vi "RTK Multiple String Capture Software.vi"() -> ()   [LabVIEW 2010]
uses:
  COM Port Control.ctl
  <vilib>/Utility/sysdir.llb/System Directory Type.ctl
  binary clusters control.ctl
  <vilib>/Instr/_visa.llb/VISA Configure Serial Port (Instr).vi
panel:
  out "shutdown blocker":bool
  in  "Tab Control":T1(tab)
  in  "Update setup":bool
  in  "stop":bool
  in  "Base File Path":path caption="Base File Path (Destination that all RCVR files will be saved in)"
  in  "Time between samples (seconds)":u32=5 min=1 max=600 step=1
  in  "Number of hours To Collect before starting new file":u16=1 min=1 max=24 step=1
  in  "UPDT COM 1":bool
  in  "Use RCVR 1":bool caption="Use RCVR"
  in  "Name of RCVR 1":string="RCVR 1" caption="Name of RCVR"
  in  "COM Port 1":T2={"flow control"=0, "COM Port"="", "parity"=enum."None", "data bits"=8, "baud rate"=9600} {"data bits" min=5 max=8 step=1; "flow control" items=["None", "XON/XOFF", "RTS/CTS", "XON/XOFF & RTS/CTS", "DTR/DSR", "XON/XOFF & DTR/DSR"]}
  out "Last 10 RCVR 1":string[](array[string])
  in  "Name of RCVR 2":string="RCVR 2" caption="Name of RCVR"
  in  "UPDT COM 2":bool
  out "Last 10 RCVR 2":string[](array[string])
  in  "COM Port 2":T2={"flow control"=0, "COM Port"="", "parity"=enum."None", "data bits"=8, "baud rate"=9600} {"data bits" min=5 max=8 step=1; "flow control" items=["None", "XON/XOFF", "RTS/CTS", "XON/XOFF & RTS/CTS", "DTR/DSR", "XON/XOFF & DTR/DSR"]}
  in  "Use RCVR 2":bool caption="Use RCVR"
  in  "Name of RCVR 3":string="RCVR 3" caption="Name of RCVR"
  in  "UPDT COM 3":bool
  out "Last 10 RCVR 3":string[](array[string])
  in  "COM Port 3":T2={"flow control"=0, "COM Port"="", "parity"=enum."None", "data bits"=8, "baud rate"=9600} {"data bits" min=5 max=8 step=1; "flow control" items=["None", "XON/XOFF", "RTS/CTS", "XON/XOFF & RTS/CTS", "DTR/DSR", "XON/XOFF & DTR/DSR"]}
  in  "Use RCVR 3":bool caption="Use RCVR"
  in  "Name of RCVR 4":string="RCVR 4" caption="Name of RCVR"
  in  "UPDT COM 4":bool
  out "Last 10 RCVR 4":string[](array[string])
  in  "COM Port 4":T2={"flow control"=0, "COM Port"="", "parity"=enum."None", "data bits"=8, "baud rate"=9600} {"data bits" min=5 max=8 step=1; "flow control" items=["None", "XON/XOFF", "RTS/CTS", "XON/XOFF & RTS/CTS", "DTR/DSR", "XON/XOFF & DTR/DSR"]}
  in  "Use RCVR 4":bool caption="Use RCVR"
  in  "Name of RCVR 5":string="RCVR 5" caption="Name of RCVR"
  in  "UPDT COM 5":bool
  out "Last 10 RCVR 5":string[](array[string])
  in  "COM Port 5":T2={"flow control"=0, "COM Port"="", "parity"=enum."None", "data bits"=8, "baud rate"=9600} {"data bits" min=5 max=8 step=1; "flow control" items=["None", "XON/XOFF", "RTS/CTS", "XON/XOFF & RTS/CTS", "DTR/DSR", "XON/XOFF & DTR/DSR"]}
  in  "Use RCVR 5":bool caption="Use RCVR"
  in  "Name of RCVR 6":string="RCVR 6" caption="Name of RCVR"
  in  "UPDT COM 6":bool
  out "Last 10 RCVR 6":string[](array[string])
  in  "COM Port 6":T2={"flow control"=0, "COM Port"="", "parity"=enum."None", "data bits"=8, "baud rate"=9600} {"data bits" min=5 max=8 step=1; "flow control" items=["None", "XON/XOFF", "RTS/CTS", "XON/XOFF & RTS/CTS", "DTR/DSR", "XON/XOFF & DTR/DSR"]}
  in  "Use RCVR 6":bool caption="Use RCVR"
  in  "Name of RCVR 7":string="RCVR 7" caption="Name of RCVR"
  in  "UPDT COM 7":bool
  out "Last 10 RCVR 7":string[](array[string])
  in  "COM Port 7":T2={"flow control"=0, "COM Port"="", "parity"=enum."None", "data bits"=8, "baud rate"=9600} {"data bits" min=5 max=8 step=1; "flow control" items=["None", "XON/XOFF", "RTS/CTS", "XON/XOFF & RTS/CTS", "DTR/DSR", "XON/XOFF & DTR/DSR"]}
  in  "Use RCVR 7":bool caption="Use RCVR"
  in  "Name of RCVR 8":string="RCVR 8" caption="Name of RCVR"
  in  "UPDT COM 8":bool
  out "Last 10 RCVR 8":string[](array[string])
  in  "COM Port 8":T2={"flow control"=0, "COM Port"="", "parity"=enum."None", "data bits"=8, "baud rate"=9600} {"data bits" min=5 max=8 step=1; "flow control" items=["None", "XON/XOFF", "RTS/CTS", "XON/XOFF & RTS/CTS", "DTR/DSR", "XON/XOFF & DTR/DSR"]}
  in  "Use RCVR 8":bool caption="Use RCVR"
  in  "Name of RCVR 9":string="RCVR 9" caption="Name of RCVR"
  in  "UPDT COM 9":bool
  out "Last 10 RCVR 9":string[](array[string])
  in  "COM Port 9":T2={"flow control"=0, "COM Port"="", "parity"=enum."None", "data bits"=8, "baud rate"=9600} {"data bits" min=5 max=8 step=1; "flow control" items=["None", "XON/XOFF", "RTS/CTS", "XON/XOFF & RTS/CTS", "DTR/DSR", "XON/XOFF & DTR/DSR"]}
  in  "Use RCVR 9":bool caption="Use RCVR"
  in  "Name of RCVR 10":string="RCVR 10" caption="Name of RCVR"
  in  "UPDT COM 10":bool
  out "Last 10 RCVR 10":string[](array[string])
  in  "COM Port 10":T2={"flow control"=0, "COM Port"="", "parity"=enum."None", "data bits"=8, "baud rate"=9600} {"data bits" min=5 max=8 step=1; "flow control" items=["None", "XON/XOFF", "RTS/CTS", "XON/XOFF & RTS/CTS", "DTR/DSR", "XON/XOFF & DTR/DSR"]}
  in  "Use RCVR 10":bool caption="Use RCVR"
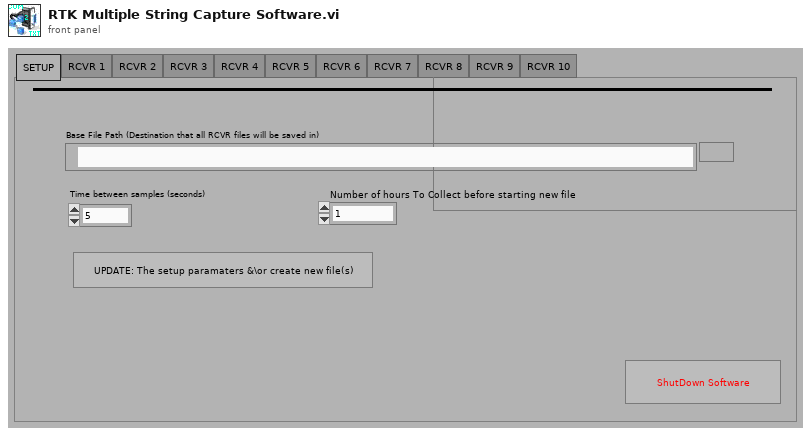
[diagram p1: front panel]
types:
  T1 = enum32{"SETUP", "RCVR 1", "RCVR 2", "RCVR 3", "RCVR 4", "RCVR 5", "RCVR 6", "RCVR 7", "RCVR 8", "RCVR 9", "RCVR 10"}
  T2 = typedef "COM Port Control.ctl" = cluster{"flow control":u16, "COM Port":refnum<visa-resource-name>, "parity":enum16{"None", "Odd", "Even", "Mark", "Space"}, "data bits":u16, "baud rate":u32}
  T3 = typedef "binary clusters control.ctl" = cluster{"setup save cluster":cluster{"Base File Path":path, "Time between samples (seconds)":u32, "Number of hours To Collect before starting new file ":u16}, "RCVR1 Save Cluster":cluster{"Use RCVR 1":bool, "COM Port 1":T2, "Name of RCVR 1":string}, "RCVR2 Save cluster":cluster{"Use RCVR 2":bool, "COM Port 2":T2, "Name of RCVR 2":string}, "RCVR3 Save Cluster":cluster{"Use RCVR 3":bool, "Name of RCVR 3":string, "COM Port 3":T2}, "RCVR4 Save Cluster":cluster{"Use RCVR 4":bool, "Name of RCVR 4":string, "COM Port 4":T2}, "RCVR5 Save Cluster":cluster{"Use RCVR 5":bool, "Name of RCVR 5":string, "COM Port 5":T2}, "RCVR6 Save Cluster":cluster{"Use RCVR 6":bool, "Name of RCVR 6":string, "COM Port 6":T2}, "RCVR7 Save Cluster":cluster{"Use RCVR 7":bool, "Name of RCVR 7":string, "COM Port 7":T2}, "RCVR8 Save Cluster":cluster{"Use RCVR 8":bool, "Name of RCVR 8":string, "COM Port 8":T2}, "RCVR9 Save Cluster":cluster{"Use RCVR 9":bool, "Name of RCVR 9":string, "COM Port 9":T2}, "RCVR10 Save Cluster":cluster{"Use RCVR 10":bool, "Name of RCVR 10":string, "COM Port 10":T2}}
  T4 = cluster{"File Path Notify":refnum<notifier>, "Time smpl notify":refnum<notifier>, "Update notify":refnum<notifier>, "shutdown notify":refnum<notifier>}
  T5 = enum16{"big-endian, network order", "native, host order", "little-endian"}
  T6 = typedef "System Directory Type.ctl" = i32
  T7 = cluster{"Base File Path":path, "Time between samples (seconds)":u32, "Number of hours To Collect before starting new file ":u16}
  T8 = cluster{"Use RCVR 1":bool, "COM Port 1":T2, "Name of RCVR 1":string}
  T9 = cluster{"Use RCVR 2":bool, "COM Port 2":T2, "Name of RCVR 2":string}
  T10 = cluster{"Use RCVR 3":bool, "Name of RCVR 3":string, "COM Port 3":T2}
  T11 = cluster{"Use RCVR 5":bool, "Name of RCVR 5":string, "COM Port 5":T2}
  T12 = cluster{"Use RCVR 6":bool, "Name of RCVR 6":string, "COM Port 6":T2}
  T13 = cluster{"Use RCVR 10":bool, "Name of RCVR 10":string, "COM Port 10":T2}
  T14 = cluster{"Use RCVR 7":bool, "Name of RCVR 7":string, "COM Port 7":T2}
  T15 = cluster{"Use RCVR 9":bool, "Name of RCVR 9":string, "COM Port 9":T2}
  T16 = cluster{"Use RCVR 8":bool, "Name of RCVR 8":string, "COM Port 8":T2}
  T17 = cluster{"Use RCVR 4":bool, "Name of RCVR 4":string, "COM Port 4":T2}
  T18 = enum32{"invalid app kind", "Development System", "Run Time System", "Student Edition", "Embedded LabVIEW", "Evaluation", "Custom"}
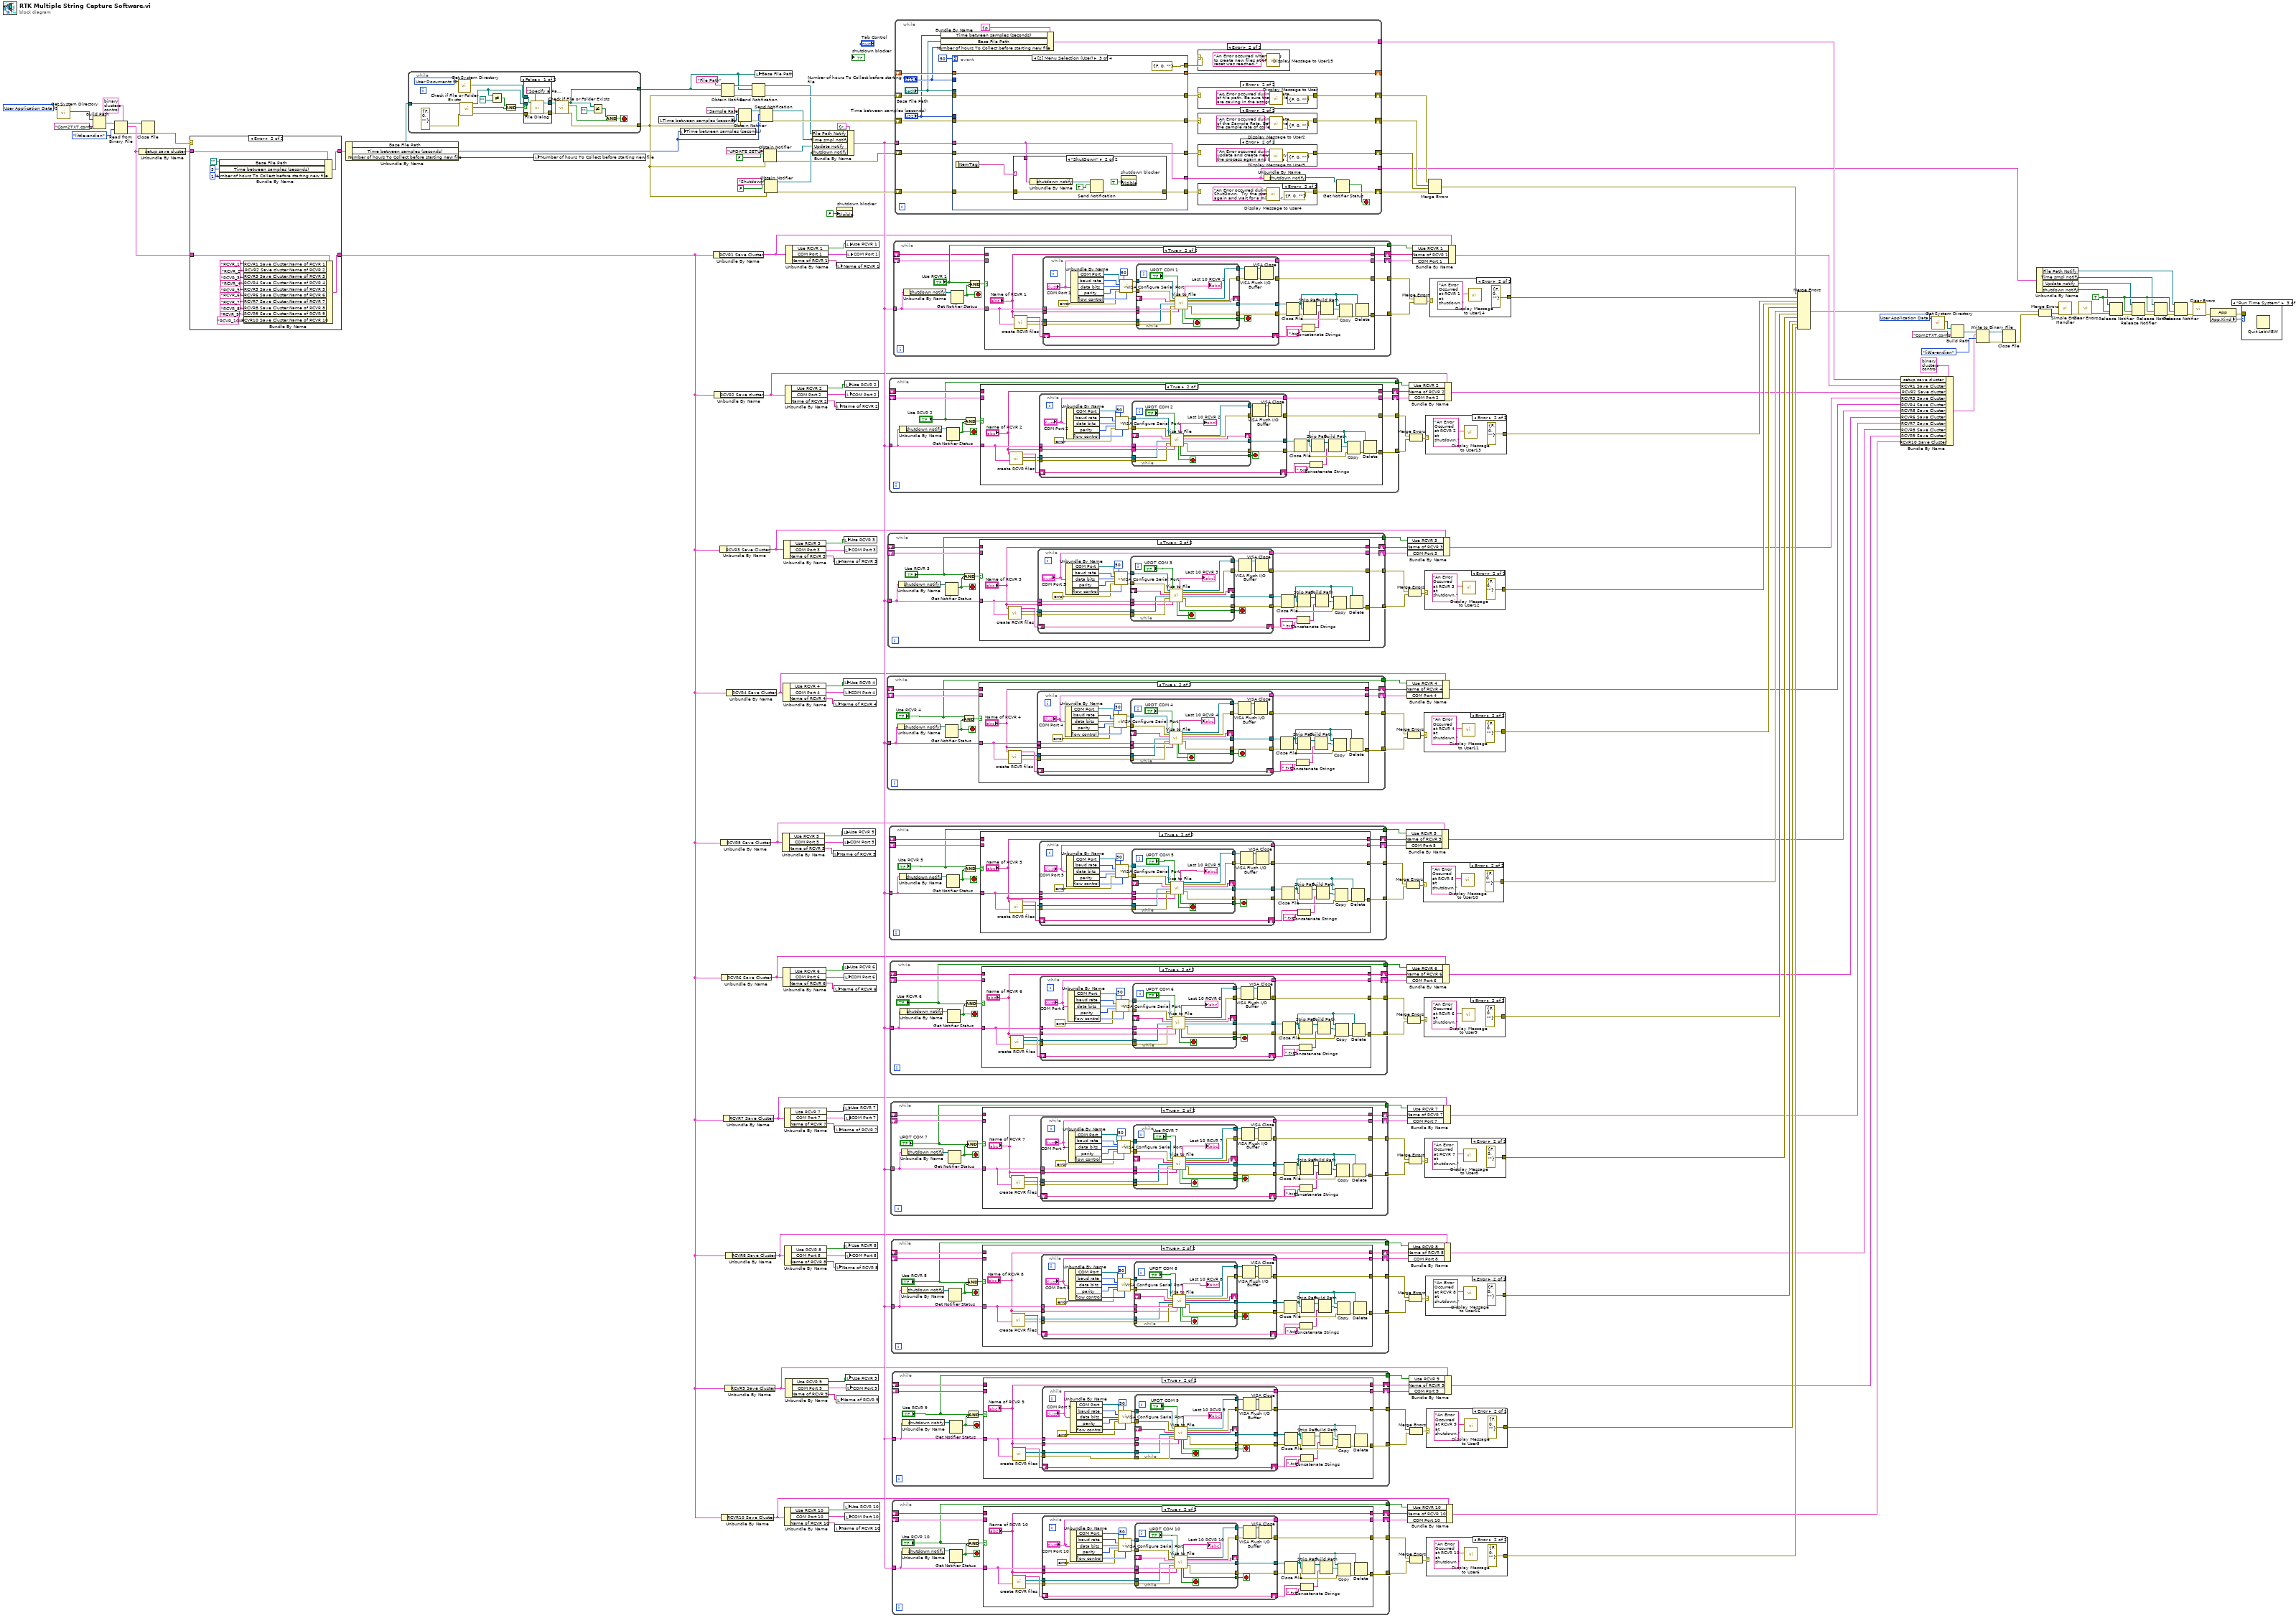
[diagram p0: block diagram]
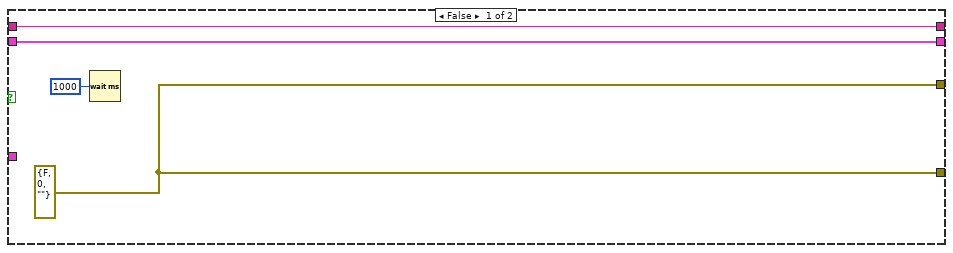
[diagram p4: hidden frame]
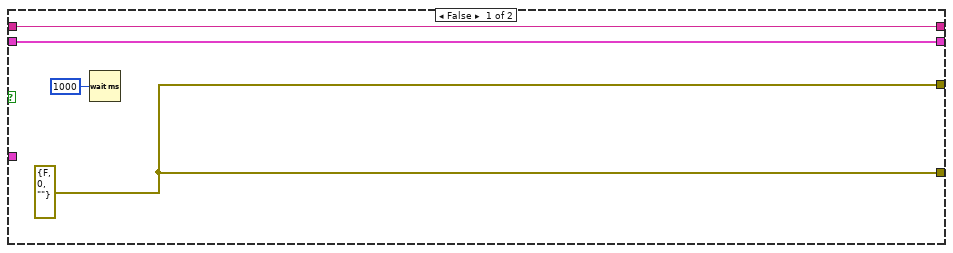
[diagram p6: hidden frame]
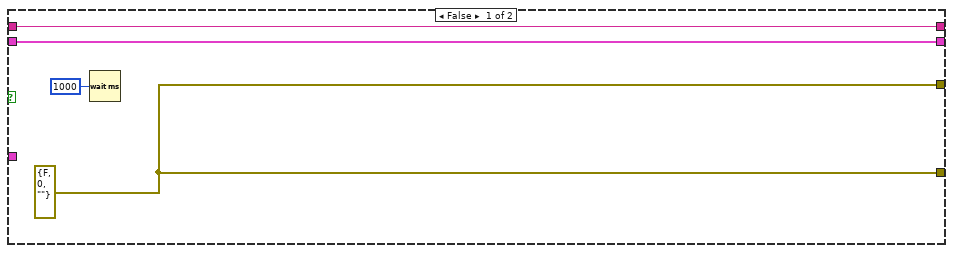
[diagram p8: hidden frame]
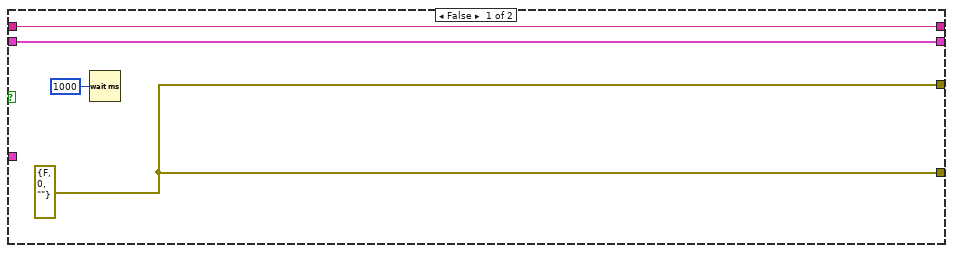
[diagram p10: hidden frame]
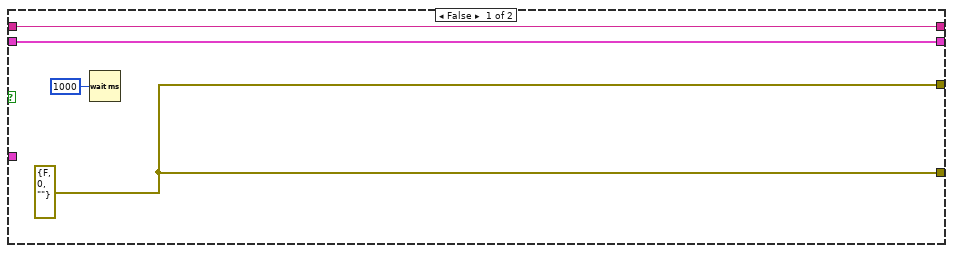
[diagram p12: hidden frame]
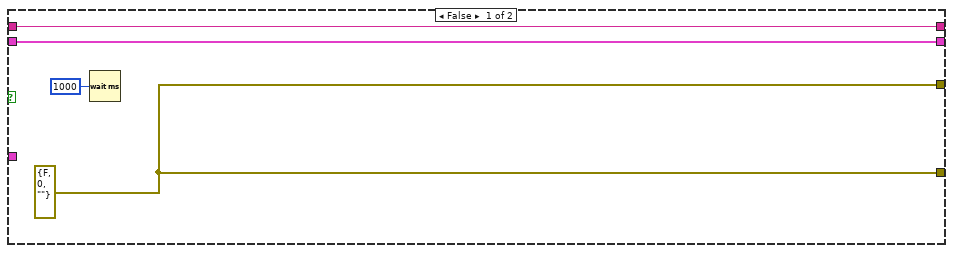
[diagram p14: hidden frame]
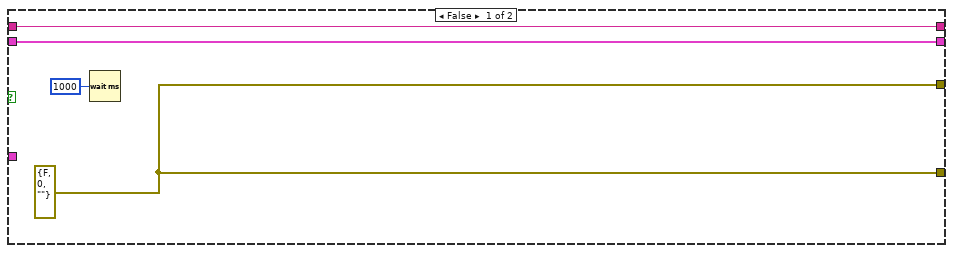
[diagram p16: hidden frame]
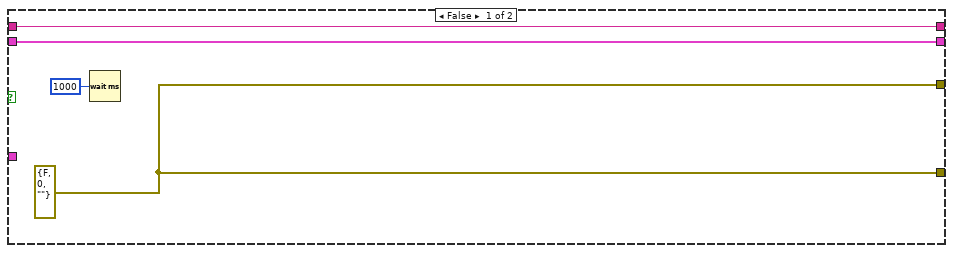
[diagram p18: hidden frame]
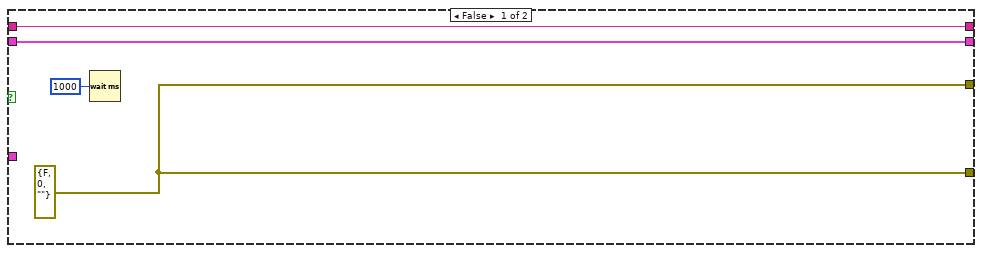
[diagram p20: hidden frame]
diagram:
  w150 = T6 3 items=["User Home"=0, "User Desktop"=1, "User Documents"=2, "User Application Data"=3, "User Preferences"=4, "User Temporary"=5, "Public Documents"=6, "Public Application Data"=7, "Public Preferences"=8, "Public Cache"=13, "System Core Libraries"=9, "System Installed Libraries"=10, "Application Files"=11, "Boot Volume Root"=12] ("system directory type")
  w157 = T6 3 items=["User Home"=0, "User Desktop"=1, "User Documents"=2, "User Application Data"=3, "User Preferences"=4, "User Temporary"=5, "Public Documents"=6, "Public Application Data"=7, "Public Preferences"=8, "Public Cache"=13, "System Core Libraries"=9, "System Installed Libraries"=10, "Application Files"=11, "Boot Volume Root"=12] ("system directory type")
  w166 = TRUE
  n1 = call <vilib>:"Get System Directory.vi"("system directory type"=w157) -> ("system directory"=w156:path)  [unwired: 10 in]
  n2 = Build Path(base path=w156, name or relative path="Com2TXT.confg") -> (appended path=w136:path)
  n3 = Read from Binary File(5:T3 {"setup save cluster"={"Base File Path"=path "", "Time between samples (seconds)"=0, "Number of hours To Collect before starting new file "=0}, "RCVR1 Save Cluster"={"Use RCVR 1"=FALSE, "COM Port 1"={"flow control"=0, "COM Port"="", "parity"=enum."None", "data bits"=0, "baud rate"=0}, "Name of RCVR 1"=""}, "RCVR2 Save cluster"={"Use RCVR 2"=FALSE, "COM Port 2"={"flow control"=0, "COM Port"="", "parity"=enum."None", "data bits"=0, "baud rate"=0}, "Name of RCVR 2"=""}, "RCVR3 Save Cluster"={"Use RCVR 3"=FALSE, "Name of RCVR 3"="", "COM Port 3"={"flow control"=0, "COM Port"="", "parity"=enum."None", "data bits"=0, "baud rate"=0}}, "RCVR4 Save Cluster"={"Use RCVR 4"=FALSE, "Name of RCVR 4"="", "COM Port 4"={"flow control"=0, "COM Port"="", "parity"=enum."None", "data bits"=0, "baud rate"=0}}, "RCVR5 Save Cluster"={"Use RCVR 5"=FALSE, "Name of RCVR 5"="", "COM Port 5"={"flow control"=0, "COM Port"="", "parity"=enum."None", "data bits"=0, "baud rate"=0}}, "RCVR6 Save Cluster"={"Use RCVR 6"=FALSE, "Name of RCVR 6"="", "COM Port 6"={"flow control"=0, "COM Port"="", "parity"=enum."None", "data bits"=0, "baud rate"=0}}, "RCVR7 Save Cluster"={"Use RCVR 7"=FALSE, "Name of RCVR 7"="", "COM Port 7"={"flow control"=0, "COM Port"="", "parity"=enum."None", "data bits"=0, "baud rate"=0}}, "RCVR8 Save Cluster"={"Use RCVR 8"=FALSE, "Name of RCVR 8"="", "COM Port 8"={"flow control"=0, "COM Port"="", "parity"=enum."None", "data bits"=0, "baud rate"=0}}, "RCVR9 Save Cluster"={"Use RCVR 9"=FALSE, "Name of RCVR 9"="", "COM Port 9"={"flow control"=0, "COM Port"="", "parity"=enum."None", "data bits"=0, "baud rate"=0}}, "RCVR10 Save Cluster"={"Use RCVR 10"=FALSE, "Name of RCVR 10"="", "COM Port 10"={"flow control"=0, "COM Port"="", "parity"=enum."None", "data bits"=0, "baud rate"=0}}} ("output cluster"), 9:T5."little-endian" ("byte order (0:big-endian, network order)"), 11:w136) -> (0:w145:errorcluster, 2:w3:T3, 3:w144:refnum<file>)  [unwired: 3 in, 1 out]
  n4 = Unbundle By Name(w3) -> ("setup save cluster"=w6:T7)
  n5 = Close File(refnum=w144, error in=w145) -> (error out=w4:errorcluster)  [unwired: 1 out]
  n6 = case shown="Error" w4 {
    tunnel: w6 -> [w195 w212]
    tunnel: [w195 w211] -> w5
    tunnel: [w194 w208] -> w2
    tunnel: w3 -> [w194 w207]
    frame No Error {
    }
    frame Error {
      n7 = Bundle By Name(cluster=w212, "Base File Path"=path "", "Time between samples (seconds)"=u32 5, "Number of hours To Collect before starting new file"=u16 1) -> (w211:T7)
      n8 = Bundle By Name(cluster=w207, "RCVR1 Save Cluster.Name of RCVR 1"="RCVR_1", "RCVR2 Save cluster.Name of RCVR 2"="RCVR_2" ("RCVR1 Save Cluster.Name of RCVR 1"), "RCVR3 Save Cluster.Name of RCVR 3"="RCVR_3" ("RCVR1 Save Cluster.Name of RCVR 1"), "RCVR4 Save Cluster.Name of RCVR 4"="RCVR_4" ("RCVR1 Save Cluster.Name of RCVR 1"), "RCVR5 Save Cluster.Name of RCVR 5"="RCVR_5" ("RCVR1 Save Cluster.Name of RCVR 1"), "RCVR6 Save Cluster.Name of RCVR 6"="RCVR_6" ("RCVR1 Save Cluster.Name of RCVR 1"), "RCVR7 Save Cluster.Name of RCVR 7"="RCVR_7" ("RCVR1 Save Cluster.Name of RCVR 1"), "RCVR8 Save Cluster.Name of RCVR 8"="RCVR_8" ("RCVR1 Save Cluster.Name of RCVR 1"), "RCVR9 Save Cluster.Name of RCVR 9"="RCVR_9" ("RCVR1 Save Cluster.Name of RCVR 1"), "RCVR10 Save Cluster.Name of RCVR 10"="RCVR_10" ("RCVR1 Save Cluster.Name of RCVR 1")) -> (w208:T3)
    }
  }
  n9 = Unbundle By Name(w5) -> ("Base File Path"=w148:path, "Time between samples (seconds)"=w146:u32, "Number of hours To Collect before starting new file"=w147:u16)
  n10 = while {
    tunnel: [w224] -> w180
    tunnel: [w226] -> w162
    tunnel: w148 -> [w215]
    stop <- w225 stop-if-true
    w214 = T6 2 items=["User Home"=0, "User Desktop"=1, "User Documents"=2, "User Application Data"=3, "User Preferences"=4, "User Temporary"=5, "Public Documents"=6, "Public Application Data"=7, "Public Preferences"=8, "Public Cache"=13, "System Core Libraries"=9, "System Installed Libraries"=10, "Application Files"=11, "Boot Volume Root"=12] ("system directory type")
    n11 = call <vilib>:"Get System Directory.vi"("system directory type"=w214) -> ("system directory"=w213:path)  [unwired: 10 in]
    n12 = call <vilib>:"Check if File or Folder Exists.vi"("error in (no error)"=errorcluster {"status"=FALSE, "code"=0, "source"=""}, "path"=w215) -> ("error out"=w228:errorcluster, "file or folder exists?"=w218:bool, "dup path"=w217:path)  [unwired: 7 in]
    n13 = Not Equal?(x=w217, y=path "") -> (x != y?=w220:bool)
    n14 = And(x=w220, y=w218) -> (x .and. y?=w216:bool)
    n15 = case shown="False" w216 {
      tunnel: [w235 w237] -> w230
      tunnel: w217 -> [_ w237]
      tunnel: w228 -> [w234 w236]
      tunnel: [w233 w236] -> w227
      tunnel: w213 -> [w231 _]
      frame False {
        n16 = call "File Dialog"("start path"=w231, "prompt"="Specify a Path to Save RCVR .TXT files", "error in"=w234) -> ("selected path"=w235:path, "error out"=w233:errorcluster)  [unwired: 9 in, 2 out]
      }
      frame True {
      }
    }
    n17 = call <vilib>:"Check if File or Folder Exists.vi"("error in (no error)"=w227, "path"=w230) -> ("error out"=w226:errorcluster, "file or folder exists?"=w221:bool, "dup path"=w224:path)  [unwired: 7 in]
    n18 = Not Equal?(x=w224, y=path "") -> (x != y?=w222:bool)
    n19 = And(x=w222, y=w221) -> (x .and. y?=w225:bool)
  }
  n20 = local write "Number of hours To Collect before starting new file"(w147) -> ()
  n21 = local read "Time between samples (seconds)"() -> (w184:u32)
  n22 = local write "Time between samples (seconds)"(w146) -> ()
  n23 = Unbundle By Name(w2) -> ("RCVR1 Save Cluster"=w18:T8)
  n24 = Unbundle By Name(w2) -> ("RCVR2 Save cluster"=w17:T9)
  n25 = Unbundle By Name(w2) -> ("RCVR3 Save Cluster"=w16:T10)
  n26 = Unbundle By Name(w2) -> ("RCVR5 Save Cluster"=w14:T11)
  n27 = Obtain Notifier(name (unnamed)="File Path", notification data type=w180, error in (no error)=w162) -> (notifier out=w183:refnum<notifier>, error out=w182:errorcluster)  [unwired: 1 in, 1 out]
  n28 = Unbundle By Name(w2) -> ("RCVR6 Save Cluster"=w13:T12)
  n29 = Unbundle By Name(w2) -> ("RCVR10 Save Cluster"=w9:T13)
  n30 = Unbundle By Name(w2) -> ("RCVR7 Save Cluster"=w12:T14)
  n31 = Unbundle By Name(w2) -> ("RCVR9 Save Cluster"=w10:T15)
  n32 = Unbundle By Name(w2) -> ("RCVR8 Save Cluster"=w11:T16)
  n33 = Unbundle By Name(w2) -> ("RCVR4 Save Cluster"=w15:T17)
  n34 = Obtain Notifier(name (unnamed)="Sample Rate", notification data type=w184, error in (no error)=w162) -> (notifier out=w177:refnum<notifier>, error out=w178:errorcluster)  [unwired: 1 in, 1 out]
  n35 = Send Notification(notification=w180, notifier=w183, error in (no error)=w182) -> (notifier out=w133:refnum<notifier>, error out=w181:errorcluster)
  n36 = local write "Base File Path"(w180) -> ()
  n37 = Send Notification(notification=w146, notifier=w177, error in (no error)=w178) -> (notifier out=w132:refnum<notifier>, error out=w179:errorcluster)
  n38 = Obtain Notifier(name (unnamed)="UPDATE SETUP", notification data type=FALSE, error in (no error)=w162) -> (notifier out=w131:refnum<notifier>, error out=w188:errorcluster)  [unwired: 1 in, 1 out]
  n39 = Obtain Notifier(name (unnamed)="Shutdown", notification data type=FALSE, error in (no error)=w162) -> (notifier out=w130:refnum<notifier>, error out=w191:errorcluster)  [unwired: 1 in, 1 out]
  n40 = Unbundle By Name(w14) -> ("Use RCVR 5"=w91:bool, "COM Port 5"=w90:T2, "Name of RCVR 5"=w89:string)
  n41 = Unbundle By Name(w15) -> ("Use RCVR 4"=w105:bool, "COM Port 4"=w106:T2, "Name of RCVR 4"=w107:string)
  n42 = Unbundle By Name(w13) -> ("Use RCVR 6"=w85:bool, "COM Port 6"=w86:T2, "Name of RCVR 6"=w87:string)
  n43 = Unbundle By Name(w16) -> ("Use RCVR 3"=w110:bool, "COM Port 3"=w109:T2, "Name of RCVR 3"=w108:string)
  n44 = Unbundle By Name(w12) -> ("Use RCVR 7"=w71:bool, "COM Port 7"=w70:T2, "Name of RCVR 7"=w69:string)
  n45 = Unbundle By Name(w9) -> ("Use RCVR 10"=w45:bool, "COM Port 10"=w46:T2, "Name of RCVR 10"=w47:string)
  n46 = Unbundle By Name(w11) -> ("Use RCVR 8"=w66:bool, "COM Port 8"=w67:T2, "Name of RCVR 8"=w68:string)
  n47 = Unbundle By Name(w17) -> ("Use RCVR 2"=w21:bool, "COM Port 2"=w20:T2, "Name of RCVR 2"=w19:string)
  n48 = Unbundle By Name(w10) -> ("Use RCVR 9"=w51:bool, "COM Port 9"=w50:T2, "Name of RCVR 9"=w49:string)
  n49 = Unbundle By Name(w18) -> ("Use RCVR 1"=w24:bool, "COM Port 1"=w23:T2, "Name of RCVR 1"=w22:string)
  n50 = Bundle By Name(cluster=T4 {"File Path Notify"=refnum, "Time smpl notify"=refnum, "Update notify"=refnum, "shutdown notify"=refnum} ("Notifiers"), "File Path Notify"=w133, "Time smpl notify"=w132, "Update notify"=w131, "shutdown notify"=w130) -> (w38:T4)
  n51 = local write "Name of RCVR 5"(w89) -> ()
  n52 = local write "Name of RCVR 4"(w107) -> ()
  n53 = local write "Name of RCVR 6"(w87) -> ()
  n54 = local write "Name of RCVR 3"(w108) -> ()
  n55 = local write "Name of RCVR 7"(w69) -> ()
  n56 = local write "Name of RCVR 10"(w47) -> ()
  n57 = local write "Name of RCVR 8"(w68) -> ()
  n58 = local write "Name of RCVR 2"(w19) -> ()
  n59 = local write "Name of RCVR 9"(w49) -> ()
  n60 = local write "Name of RCVR 1"(w22) -> ()
  n61 = property on="shutdown blocker" class="Bool (strict)"("Visible"=FALSE) -> ()  [unwired: 2 in, 2 out]
  n62 = local write "Use RCVR 5"(w91) -> ()
  n63 = local write "Use RCVR 4"(w105) -> ()
  n64 = local write "COM Port 5"(w90) -> ()
  n65 = local write "Use RCVR 6"(w85) -> ()
  n66 = local write "Use RCVR 3"(w110) -> ()
  n67 = local write "COM Port 4"(w106) -> ()
  n68 = local write "COM Port 6"(w86) -> ()
  n69 = local write "Use RCVR 7"(w71) -> ()
  n70 = local write "Use RCVR 10"(w45) -> ()
  n71 = local write "COM Port 3"(w109) -> ()
  n72 = local write "Use RCVR 8"(w66) -> ()
  n73 = local write "Use RCVR 2"(w21) -> ()
  n74 = local write "COM Port 7"(w70) -> ()
  n75 = local write "COM Port 10"(w46) -> ()
  n76 = local write "COM Port 8"(w67) -> ()
  n77 = local write "Use RCVR 9"(w51) -> ()
  n78 = local write "Use RCVR 1"(w24) -> ()
  n79 = local write "COM Port 2"(w20) -> ()
  n80 = local write "COM Port 9"(w50) -> ()
  n81 = local write "COM Port 1"(w23) -> ()
  n82 = while {
    tunnel: [w247] -> w101
    tunnel: [w248] -> w100
    tunnel: ["Use RCVR 4"] -> w102
    shift-right: [w244] -> w103
    shift-left: _ -> [w243]
    shift-right: [w242] -> w104
    shift-left: _ -> [w240]
    tunnel: w38 -> [w239]
    stop <- w245 stop-if-true
    n83 = Unbundle By Name(w239) -> ("shutdown notify"=w241:refnum<notifier>)
    n84 = Get Notifier Status(notifier=w241) -> (current notification=w245:bool)  [unwired: 1 in, 4 out]
    n85 = Compound Arithmetic op=AND("Use RCVR 4", invert w245) -> (w246:bool)
    n86 = case shown="True" w246 {
      tunnel: [w251 w268] -> w248
      tunnel: [w251 w262] -> w247
      tunnel: [w250 "Name of RCVR 4"] -> w244
      tunnel: w243 -> [w250 _]
      tunnel: [w249 w255] -> w242
      tunnel: w240 -> [w249 _]
      tunnel: w239 -> [_ w254]
      frame False {
        w251 = errorcluster {"status"=FALSE, "code"=0, "source"=""} ("error in (no error)")
        n87 = Wait (ms)(milliseconds to wait=u32 1000) -> ()  [unwired: 1 out]
      }
      frame True {
        n88 = call "create RCVR files.vi"("Notifiers"=w254, "Name of RCVR 1"="Name of RCVR 4") -> ("error out"=w256:errorcluster, "refnum out"=w257:refnum<file>, "Name of file out"=w258:string)  [unwired: 7 in]
        n89 = while {
          tunnel: w257 -> [w293]
          tunnel: w256 -> [w292]
          tunnel: [w284] -> w270
          tunnel: [w276] -> w269
          tunnel: [w282] -> w268
          shift-right: [w274] -> w261
          shift-left: w258 -> [w274]
          tunnel: ["COM Port 4"] -> w255
          tunnel: w254 -> [w273]
          tunnel: "Name of RCVR 4" -> [w271]
          stop <- w275 stop-if-true
          n90 = Unbundle By Name("COM Port 4") -> ("COM Port"=w289:refnum<visa-resource-name>, "baud rate"=w288:u32, "data bits"=w287:u16, "parity"=w286:enum16{"None", "Odd", "Even", "Mark", "Space"}, "flow control"=w285:u16)
          n91 = call-poly "VISA Configure Serial Port"("VISA resource name"=w289, "timeout (10sec)"=u32 50, "baud rate (9600)"=w288, "data bits (8)"=w287, "parity (0:none)"=w286, "error in (no error)"=errorcluster {"status"=FALSE, "code"=0, "source"=""}, "flow control (0:none)"=w285) -> ("VISA resource name out"=w291:refnum<visa-resource-name>, "error out"=w290:errorcluster)  [unwired: 7 in]
          n92 = while {
            tunnel: [w305] -> w278
            tunnel: w293 -> [w298]
            tunnel: w292 -> [w297]
            tunnel: w291 -> [w309]
            tunnel: [w303] -> w284
            tunnel: [w302] -> w276
            tunnel: [w301] -> w275
            shift-right: [w306] -> _
            shift-left: _ -> [w307]
            tunnel: w290 -> [w308]
            tunnel: [w304] -> w279
            tunnel: w273 -> [w299]
            tunnel: w271 -> [w294]
            stop <- w300 stop-if-true
            n93 = call "Visa to File.vi"("VISA resource name in"=w309, "Visa Error"=w308, "Array in from shift reg"=w307, "File data refnum"=w298, "File handle Error"=w297, "Notifiers"=w299, "UPDT COM switch"="UPDT COM 4", "Name of RCVR 1"=w294) -> ("End Visa Loop"=w300:bool, "Last 10 RCVR 1"=→"Last 10 RCVR 4":string[], "End File Loop"=w301:bool, "VISA resource name out"=w305:refnum<visa-resource-name>, "Visa error out"=w304:errorcluster, "Array out to shift reg"=w306:string[], "File data refnum out"=w303:refnum<file>, "File Error out"=w302:errorcluster)  [unwired: 4 in]
          }
          n94 = VISA Flush I/O Buffer(VISA resource name=w278, error in (no error)=w279) -> (VISA resource name out=w281:refnum<visa-resource-name>, error out=w280:errorcluster)  [unwired: 1 in]
          n95 = VISA Close(VISA resource name=w281, error in (no error)=w280) -> (error out=w282:errorcluster)
        }
        n96 = Close File(refnum=w270, error in=w269) -> (path=w263:path, error out=w264:errorcluster)
        n97 = Concatenate Strings(w261, ".txt" ("string")) -> (w259:string)
        n98 = Strip Path(path=w263) -> (stripped path=w266:path)  [unwired: 1 out]
        n99 = Build Path(base path=w266, name or relative path=w259) -> (appended path=w267:path)
        n100 = Copy(8:w264, 10:w267, 11:w263) -> (0:w265:errorcluster)  [unwired: 2 in, 2 out]
        n101 = Delete(path (use dialog)=w263, error in=w265) -> (error out=w262:errorcluster)  [unwired: 3 in, 2 out]
      }
    }
  }
  n102 = while {
    tunnel: [w319] -> w115
    tunnel: [w320] -> w116
    tunnel: ["Use RCVR 3"] -> w114
    shift-right: [w316] -> w113
    shift-left: _ -> [w315]
    shift-right: [w314] -> w112
    shift-left: _ -> [w312]
    tunnel: w38 -> [w311]
    stop <- w317 stop-if-true
    n103 = Unbundle By Name(w311) -> ("shutdown notify"=w313:refnum<notifier>)
    n104 = Get Notifier Status(notifier=w313) -> (current notification=w317:bool)  [unwired: 1 in, 4 out]
    n105 = Compound Arithmetic op=AND("Use RCVR 3", invert w317) -> (w318:bool)
    n106 = case shown="True" w318 {
      tunnel: [w323 w340] -> w320
      tunnel: [w323 w334] -> w319
      tunnel: [w322 "Name of RCVR 3"] -> w316
      tunnel: w315 -> [w322 _]
      tunnel: [w321 w327] -> w314
      tunnel: w312 -> [w321 _]
      tunnel: w311 -> [_ w326]
      frame False {
        w323 = errorcluster {"status"=FALSE, "code"=0, "source"=""} ("error in (no error)")
        n107 = Wait (ms)(milliseconds to wait=u32 1000) -> ()  [unwired: 1 out]
      }
      frame True {
        n108 = call "create RCVR files.vi"("Notifiers"=w326, "Name of RCVR 1"="Name of RCVR 3") -> ("error out"=w328:errorcluster, "refnum out"=w329:refnum<file>, "Name of file out"=w330:string)  [unwired: 7 in]
        n109 = while {
          tunnel: w329 -> [w365]
          tunnel: w328 -> [w364]
          tunnel: [w356] -> w342
          tunnel: [w348] -> w341
          tunnel: [w354] -> w340
          shift-right: [w346] -> w333
          shift-left: w330 -> [w346]
          tunnel: ["COM Port 3"] -> w327
          tunnel: w326 -> [w345]
          tunnel: "Name of RCVR 3" -> [w343]
          stop <- w347 stop-if-true
          n110 = Unbundle By Name("COM Port 3") -> ("COM Port"=w361:refnum<visa-resource-name>, "baud rate"=w360:u32, "data bits"=w359:u16, "parity"=w358:enum16{"None", "Odd", "Even", "Mark", "Space"}, "flow control"=w357:u16)
          n111 = call-poly "VISA Configure Serial Port"("VISA resource name"=w361, "timeout (10sec)"=u32 50, "baud rate (9600)"=w360, "data bits (8)"=w359, "parity (0:none)"=w358, "error in (no error)"=errorcluster {"status"=FALSE, "code"=0, "source"=""}, "flow control (0:none)"=w357) -> ("VISA resource name out"=w363:refnum<visa-resource-name>, "error out"=w362:errorcluster)  [unwired: 7 in]
          n112 = while {
            tunnel: [w377] -> w350
            tunnel: w365 -> [w370]
            tunnel: w364 -> [w369]
            tunnel: w363 -> [w381]
            tunnel: [w375] -> w356
            tunnel: [w374] -> w348
            tunnel: [w373] -> w347
            shift-right: [w378] -> _
            shift-left: _ -> [w379]
            tunnel: w362 -> [w380]
            tunnel: [w376] -> w351
            tunnel: w345 -> [w371]
            tunnel: w343 -> [w366]
            stop <- w372 stop-if-true
            n113 = call "Visa to File.vi"("VISA resource name in"=w381, "Visa Error"=w380, "Array in from shift reg"=w379, "File data refnum"=w370, "File handle Error"=w369, "Notifiers"=w371, "UPDT COM switch"="UPDT COM 3", "Name of RCVR 1"=w366) -> ("End Visa Loop"=w372:bool, "Last 10 RCVR 1"=→"Last 10 RCVR 3":string[], "End File Loop"=w373:bool, "VISA resource name out"=w377:refnum<visa-resource-name>, "Visa error out"=w376:errorcluster, "Array out to shift reg"=w378:string[], "File data refnum out"=w375:refnum<file>, "File Error out"=w374:errorcluster)  [unwired: 4 in]
          }
          n114 = VISA Flush I/O Buffer(VISA resource name=w350, error in (no error)=w351) -> (VISA resource name out=w353:refnum<visa-resource-name>, error out=w352:errorcluster)  [unwired: 1 in]
          n115 = VISA Close(VISA resource name=w353, error in (no error)=w352) -> (error out=w354:errorcluster)
        }
        n116 = Close File(refnum=w342, error in=w341) -> (path=w335:path, error out=w336:errorcluster)
        n117 = Concatenate Strings(w333, ".txt" ("string")) -> (w331:string)
        n118 = Strip Path(path=w335) -> (stripped path=w338:path)  [unwired: 1 out]
        n119 = Build Path(base path=w338, name or relative path=w331) -> (appended path=w339:path)
        n120 = Copy(8:w336, 10:w339, 11:w335) -> (0:w337:errorcluster)  [unwired: 2 in, 2 out]
        n121 = Delete(path (use dialog)=w335, error in=w337) -> (error out=w334:errorcluster)  [unwired: 3 in, 2 out]
      }
    }
  }
  n122 = while {
    tunnel: [w391] -> w121
    tunnel: [w392] -> w120
    tunnel: ["Use RCVR 2"] -> w122
    shift-right: [w388] -> w123
    shift-left: _ -> [w387]
    shift-right: [w386] -> w124
    shift-left: _ -> [w384]
    tunnel: w38 -> [w382]
    stop <- w389 stop-if-true
    n123 = Unbundle By Name(w382) -> ("shutdown notify"=w385:refnum<notifier>)
    n124 = Get Notifier Status(notifier=w385) -> (current notification=w389:bool)  [unwired: 1 in, 4 out]
    n125 = Compound Arithmetic op=AND("Use RCVR 2", invert w389) -> (w390:bool)
    n126 = case shown="True" w390 {
      tunnel: [w395 w412] -> w392
      tunnel: [w395 w406] -> w391
      tunnel: [w394 "Name of RCVR 2"] -> w388
      tunnel: w387 -> [w394 _]
      tunnel: [w393 w399] -> w386
      tunnel: w384 -> [w393 _]
      tunnel: w382 -> [_ w398]
      frame False {
        w395 = errorcluster {"status"=FALSE, "code"=0, "source"=""} ("error in (no error)")
        n127 = Wait (ms)(milliseconds to wait=u32 1000) -> ()  [unwired: 1 out]
      }
      frame True {
        n128 = call "create RCVR files.vi"("Notifiers"=w398, "Name of RCVR 1"="Name of RCVR 2") -> ("error out"=w400:errorcluster, "refnum out"=w401:refnum<file>, "Name of file out"=w402:string)  [unwired: 7 in]
        n129 = while {
          tunnel: w401 -> [w437]
          tunnel: w400 -> [w436]
          tunnel: [w428] -> w414
          tunnel: [w420] -> w413
          tunnel: [w426] -> w412
          shift-right: [w418] -> w405
          shift-left: w402 -> [w418]
          tunnel: ["COM Port 2"] -> w399
          tunnel: w398 -> [w417]
          tunnel: "Name of RCVR 2" -> [w415]
          stop <- w419 stop-if-true
          n130 = Unbundle By Name("COM Port 2") -> ("COM Port"=w433:refnum<visa-resource-name>, "baud rate"=w432:u32, "data bits"=w431:u16, "parity"=w430:enum16{"None", "Odd", "Even", "Mark", "Space"}, "flow control"=w429:u16)
          n131 = call-poly "VISA Configure Serial Port"("VISA resource name"=w433, "timeout (10sec)"=u32 50, "baud rate (9600)"=w432, "data bits (8)"=w431, "parity (0:none)"=w430, "error in (no error)"=errorcluster {"status"=FALSE, "code"=0, "source"=""}, "flow control (0:none)"=w429) -> ("VISA resource name out"=w435:refnum<visa-resource-name>, "error out"=w434:errorcluster)  [unwired: 7 in]
          n132 = while {
            tunnel: [w449] -> w422
            tunnel: w437 -> [w442]
            tunnel: w436 -> [w441]
            tunnel: w435 -> [w453]
            tunnel: [w447] -> w428
            tunnel: [w446] -> w420
            tunnel: [w445] -> w419
            shift-right: [w450] -> _
            shift-left: _ -> [w451]
            tunnel: w434 -> [w452]
            tunnel: [w448] -> w423
            tunnel: w417 -> [w443]
            tunnel: w415 -> [w438]
            stop <- w444 stop-if-true
            n133 = call "Visa to File.vi"("VISA resource name in"=w453, "Visa Error"=w452, "Array in from shift reg"=w451, "File data refnum"=w442, "File handle Error"=w441, "Notifiers"=w443, "UPDT COM switch"="UPDT COM 2", "Name of RCVR 1"=w438) -> ("End Visa Loop"=w444:bool, "Last 10 RCVR 1"=→"Last 10 RCVR 2":string[], "End File Loop"=w445:bool, "VISA resource name out"=w449:refnum<visa-resource-name>, "Visa error out"=w448:errorcluster, "Array out to shift reg"=w450:string[], "File data refnum out"=w447:refnum<file>, "File Error out"=w446:errorcluster)  [unwired: 4 in]
          }
          n134 = VISA Flush I/O Buffer(VISA resource name=w422, error in (no error)=w423) -> (VISA resource name out=w425:refnum<visa-resource-name>, error out=w424:errorcluster)  [unwired: 1 in]
          n135 = VISA Close(VISA resource name=w425, error in (no error)=w424) -> (error out=w426:errorcluster)
        }
        n136 = Close File(refnum=w414, error in=w413) -> (path=w407:path, error out=w408:errorcluster)
        n137 = Concatenate Strings(w405, ".txt" ("string")) -> (w403:string)
        n138 = Strip Path(path=w407) -> (stripped path=w410:path)  [unwired: 1 out]
        n139 = Build Path(base path=w410, name or relative path=w403) -> (appended path=w411:path)
        n140 = Copy(8:w408, 10:w411, 11:w407) -> (0:w409:errorcluster)  [unwired: 2 in, 2 out]
        n141 = Delete(path (use dialog)=w407, error in=w409) -> (error out=w406:errorcluster)  [unwired: 3 in, 2 out]
      }
    }
  }
  n142 = while {
    tunnel: [w463] -> w95
    tunnel: [w464] -> w96
    tunnel: ["Use RCVR 5"] -> w94
    shift-right: [w460] -> w93
    shift-left: _ -> [w459]
    shift-right: [w458] -> w92
    shift-left: _ -> [w456]
    tunnel: w38 -> [w455]
    stop <- w461 stop-if-true
    n143 = Unbundle By Name(w455) -> ("shutdown notify"=w457:refnum<notifier>)
    n144 = Get Notifier Status(notifier=w457) -> (current notification=w461:bool)  [unwired: 1 in, 4 out]
    n145 = Compound Arithmetic op=AND("Use RCVR 5", invert w461) -> (w462:bool)
    n146 = case shown="True" w462 {
      tunnel: [w467 w484] -> w464
      tunnel: [w467 w478] -> w463
      tunnel: [w466 "Name of RCVR 5"] -> w460
      tunnel: w459 -> [w466 _]
      tunnel: [w465 w471] -> w458
      tunnel: w456 -> [w465 _]
      tunnel: w455 -> [_ w470]
      frame False {
        w467 = errorcluster {"status"=FALSE, "code"=0, "source"=""} ("error in (no error)")
        n147 = Wait (ms)(milliseconds to wait=u32 1000) -> ()  [unwired: 1 out]
      }
      frame True {
        n148 = call "create RCVR files.vi"("Notifiers"=w470, "Name of RCVR 1"="Name of RCVR 5") -> ("error out"=w472:errorcluster, "refnum out"=w473:refnum<file>, "Name of file out"=w474:string)  [unwired: 7 in]
        n149 = while {
          tunnel: w473 -> [w509]
          tunnel: w472 -> [w508]
          tunnel: [w500] -> w486
          tunnel: [w492] -> w485
          tunnel: [w498] -> w484
          shift-right: [w490] -> w477
          shift-left: w474 -> [w490]
          tunnel: ["COM Port 5"] -> w471
          tunnel: w470 -> [w489]
          tunnel: "Name of RCVR 5" -> [w487]
          stop <- w491 stop-if-true
          n150 = Unbundle By Name("COM Port 5") -> ("COM Port"=w505:refnum<visa-resource-name>, "baud rate"=w504:u32, "data bits"=w503:u16, "parity"=w502:enum16{"None", "Odd", "Even", "Mark", "Space"}, "flow control"=w501:u16)
          n151 = call-poly "VISA Configure Serial Port"("VISA resource name"=w505, "timeout (10sec)"=u32 50, "baud rate (9600)"=w504, "data bits (8)"=w503, "parity (0:none)"=w502, "error in (no error)"=errorcluster {"status"=FALSE, "code"=0, "source"=""}, "flow control (0:none)"=w501) -> ("VISA resource name out"=w507:refnum<visa-resource-name>, "error out"=w506:errorcluster)  [unwired: 7 in]
          n152 = while {
            tunnel: [w521] -> w494
            tunnel: w509 -> [w514]
            tunnel: w508 -> [w513]
            tunnel: w507 -> [w525]
            tunnel: [w519] -> w500
            tunnel: [w518] -> w492
            tunnel: [w517] -> w491
            shift-right: [w522] -> _
            shift-left: _ -> [w523]
            tunnel: w506 -> [w524]
            tunnel: [w520] -> w495
            tunnel: w489 -> [w515]
            tunnel: w487 -> [w510]
            stop <- w516 stop-if-true
            n153 = call "Visa to File.vi"("VISA resource name in"=w525, "Visa Error"=w524, "Array in from shift reg"=w523, "File data refnum"=w514, "File handle Error"=w513, "Notifiers"=w515, "UPDT COM switch"="UPDT COM 5", "Name of RCVR 1"=w510) -> ("End Visa Loop"=w516:bool, "Last 10 RCVR 1"=→"Last 10 RCVR 5":string[], "End File Loop"=w517:bool, "VISA resource name out"=w521:refnum<visa-resource-name>, "Visa error out"=w520:errorcluster, "Array out to shift reg"=w522:string[], "File data refnum out"=w519:refnum<file>, "File Error out"=w518:errorcluster)  [unwired: 4 in]
          }
          n154 = VISA Flush I/O Buffer(VISA resource name=w494, error in (no error)=w495) -> (VISA resource name out=w497:refnum<visa-resource-name>, error out=w496:errorcluster)  [unwired: 1 in]
          n155 = VISA Close(VISA resource name=w497, error in (no error)=w496) -> (error out=w498:errorcluster)
        }
        n156 = Close File(refnum=w486, error in=w485) -> (path=w479:path, error out=w480:errorcluster)
        n157 = Concatenate Strings(w477, ".txt" ("string")) -> (w475:string)
        n158 = Strip Path(path=w479) -> (stripped path=w482:path)  [unwired: 1 out]
        n159 = Build Path(base path=w482, name or relative path=w475) -> (appended path=w483:path)
        n160 = Copy(8:w480, 10:w483, 11:w479) -> (0:w481:errorcluster)  [unwired: 2 in, 2 out]
        n161 = Delete(path (use dialog)=w479, error in=w481) -> (error out=w478:errorcluster)  [unwired: 3 in, 2 out]
      }
    }
  }
  n162 = while {
    tunnel: [w535] -> w81
    tunnel: [w536] -> w80
    tunnel: ["Use RCVR 6"] -> w82
    shift-right: [w532] -> w83
    shift-left: _ -> [w531]
    shift-right: [w530] -> w84
    shift-left: _ -> [w528]
    tunnel: w38 -> [w527]
    stop <- w533 stop-if-true
    n163 = Unbundle By Name(w527) -> ("shutdown notify"=w529:refnum<notifier>)
    n164 = Get Notifier Status(notifier=w529) -> (current notification=w533:bool)  [unwired: 1 in, 4 out]
    n165 = Compound Arithmetic op=AND("Use RCVR 6", invert w533) -> (w534:bool)
    n166 = case shown="True" w534 {
      tunnel: [w539 w556] -> w536
      tunnel: [w539 w550] -> w535
      tunnel: [w538 "Name of RCVR 6"] -> w532
      tunnel: w531 -> [w538 _]
      tunnel: [w537 w543] -> w530
      tunnel: w528 -> [w537 _]
      tunnel: w527 -> [_ w542]
      frame False {
        w539 = errorcluster {"status"=FALSE, "code"=0, "source"=""} ("error in (no error)")
        n167 = Wait (ms)(milliseconds to wait=u32 1000) -> ()  [unwired: 1 out]
      }
      frame True {
        n168 = call "create RCVR files.vi"("Notifiers"=w542, "Name of RCVR 1"="Name of RCVR 6") -> ("error out"=w544:errorcluster, "refnum out"=w545:refnum<file>, "Name of file out"=w546:string)  [unwired: 7 in]
        n169 = while {
          tunnel: w545 -> [w581]
          tunnel: w544 -> [w580]
          tunnel: [w572] -> w558
          tunnel: [w564] -> w557
          tunnel: [w570] -> w556
          shift-right: [w562] -> w549
          shift-left: w546 -> [w562]
          tunnel: ["COM Port 6"] -> w543
          tunnel: w542 -> [w561]
          tunnel: "Name of RCVR 6" -> [w559]
          stop <- w563 stop-if-true
          n170 = Unbundle By Name("COM Port 6") -> ("COM Port"=w577:refnum<visa-resource-name>, "baud rate"=w576:u32, "data bits"=w575:u16, "parity"=w574:enum16{"None", "Odd", "Even", "Mark", "Space"}, "flow control"=w573:u16)
          n171 = call-poly "VISA Configure Serial Port"("VISA resource name"=w577, "timeout (10sec)"=u32 50, "baud rate (9600)"=w576, "data bits (8)"=w575, "parity (0:none)"=w574, "error in (no error)"=errorcluster {"status"=FALSE, "code"=0, "source"=""}, "flow control (0:none)"=w573) -> ("VISA resource name out"=w579:refnum<visa-resource-name>, "error out"=w578:errorcluster)  [unwired: 7 in]
          n172 = while {
            tunnel: [w593] -> w566
            tunnel: w581 -> [w586]
            tunnel: w580 -> [w585]
            tunnel: w579 -> [w597]
            tunnel: [w591] -> w572
            tunnel: [w590] -> w564
            tunnel: [w589] -> w563
            shift-right: [w594] -> _
            shift-left: _ -> [w595]
            tunnel: w578 -> [w596]
            tunnel: [w592] -> w567
            tunnel: w561 -> [w587]
            tunnel: w559 -> [w582]
            stop <- w588 stop-if-true
            n173 = call "Visa to File.vi"("VISA resource name in"=w597, "Visa Error"=w596, "Array in from shift reg"=w595, "File data refnum"=w586, "File handle Error"=w585, "Notifiers"=w587, "UPDT COM switch"="UPDT COM 6", "Name of RCVR 1"=w582) -> ("End Visa Loop"=w588:bool, "Last 10 RCVR 1"=→"Last 10 RCVR 6":string[], "End File Loop"=w589:bool, "VISA resource name out"=w593:refnum<visa-resource-name>, "Visa error out"=w592:errorcluster, "Array out to shift reg"=w594:string[], "File data refnum out"=w591:refnum<file>, "File Error out"=w590:errorcluster)  [unwired: 4 in]
          }
          n174 = VISA Flush I/O Buffer(VISA resource name=w566, error in (no error)=w567) -> (VISA resource name out=w569:refnum<visa-resource-name>, error out=w568:errorcluster)  [unwired: 1 in]
          n175 = VISA Close(VISA resource name=w569, error in (no error)=w568) -> (error out=w570:errorcluster)
        }
        n176 = Close File(refnum=w558, error in=w557) -> (path=w551:path, error out=w552:errorcluster)
        n177 = Concatenate Strings(w549, ".txt" ("string")) -> (w547:string)
        n178 = Strip Path(path=w551) -> (stripped path=w554:path)  [unwired: 1 out]
        n179 = Build Path(base path=w554, name or relative path=w547) -> (appended path=w555:path)
        n180 = Copy(8:w552, 10:w555, 11:w551) -> (0:w553:errorcluster)  [unwired: 2 in, 2 out]
        n181 = Delete(path (use dialog)=w551, error in=w553) -> (error out=w550:errorcluster)  [unwired: 3 in, 2 out]
      }
    }
  }
  n182 = while {
    tunnel: [w607] -> w75
    tunnel: [w608] -> w76
    tunnel: ["UPDT COM 7"] -> w74
    shift-right: [w604] -> w73
    shift-left: _ -> [w603]
    shift-right: [w602] -> w72
    shift-left: _ -> [w600]
    tunnel: w38 -> [w599]
    stop <- w605 stop-if-true
    n183 = Unbundle By Name(w599) -> ("shutdown notify"=w601:refnum<notifier>)
    n184 = Get Notifier Status(notifier=w601) -> (current notification=w605:bool)  [unwired: 1 in, 4 out]
    n185 = Compound Arithmetic op=AND("UPDT COM 7", invert w605) -> (w606:bool)
    n186 = case shown="True" w606 {
      tunnel: [w611 w628] -> w608
      tunnel: [w611 w622] -> w607
      tunnel: [w610 "Name of RCVR 7"] -> w604
      tunnel: w603 -> [w610 _]
      tunnel: [w609 w615] -> w602
      tunnel: w600 -> [w609 _]
      tunnel: w599 -> [_ w614]
      frame False {
        w611 = errorcluster {"status"=FALSE, "code"=0, "source"=""} ("error in (no error)")
        n187 = Wait (ms)(milliseconds to wait=u32 1000) -> ()  [unwired: 1 out]
      }
      frame True {
        n188 = call "create RCVR files.vi"("Notifiers"=w614, "Name of RCVR 1"="Name of RCVR 7") -> ("error out"=w616:errorcluster, "refnum out"=w617:refnum<file>, "Name of file out"=w618:string)  [unwired: 7 in]
        n189 = while {
          tunnel: w617 -> [w653]
          tunnel: w616 -> [w652]
          tunnel: [w644] -> w630
          tunnel: [w636] -> w629
          tunnel: [w642] -> w628
          shift-right: [w634] -> w621
          shift-left: w618 -> [w634]
          tunnel: ["COM Port 7"] -> w615
          tunnel: w614 -> [w633]
          tunnel: "Name of RCVR 7" -> [w631]
          stop <- w635 stop-if-true
          n190 = Unbundle By Name("COM Port 7") -> ("COM Port"=w649:refnum<visa-resource-name>, "baud rate"=w648:u32, "data bits"=w647:u16, "parity"=w646:enum16{"None", "Odd", "Even", "Mark", "Space"}, "flow control"=w645:u16)
          n191 = call-poly "VISA Configure Serial Port"("VISA resource name"=w649, "timeout (10sec)"=u32 50, "baud rate (9600)"=w648, "data bits (8)"=w647, "parity (0:none)"=w646, "error in (no error)"=errorcluster {"status"=FALSE, "code"=0, "source"=""}, "flow control (0:none)"=w645) -> ("VISA resource name out"=w651:refnum<visa-resource-name>, "error out"=w650:errorcluster)  [unwired: 7 in]
          n192 = while {
            tunnel: [w665] -> w638
            tunnel: w653 -> [w658]
            tunnel: w652 -> [w657]
            tunnel: w651 -> [w669]
            tunnel: [w663] -> w644
            tunnel: [w662] -> w636
            tunnel: [w661] -> w635
            shift-right: [w666] -> _
            shift-left: _ -> [w667]
            tunnel: w650 -> [w668]
            tunnel: [w664] -> w639
            tunnel: w633 -> [w659]
            tunnel: w631 -> [w654]
            stop <- w660 stop-if-true
            n193 = call "Visa to File.vi"("VISA resource name in"=w669, "Visa Error"=w668, "Array in from shift reg"=w667, "File data refnum"=w658, "File handle Error"=w657, "Notifiers"=w659, "UPDT COM switch"="Use RCVR 7", "Name of RCVR 1"=w654) -> ("End Visa Loop"=w660:bool, "Last 10 RCVR 1"=→"Last 10 RCVR 7":string[], "End File Loop"=w661:bool, "VISA resource name out"=w665:refnum<visa-resource-name>, "Visa error out"=w664:errorcluster, "Array out to shift reg"=w666:string[], "File data refnum out"=w663:refnum<file>, "File Error out"=w662:errorcluster)  [unwired: 4 in]
          }
          n194 = VISA Flush I/O Buffer(VISA resource name=w638, error in (no error)=w639) -> (VISA resource name out=w641:refnum<visa-resource-name>, error out=w640:errorcluster)  [unwired: 1 in]
          n195 = VISA Close(VISA resource name=w641, error in (no error)=w640) -> (error out=w642:errorcluster)
        }
        n196 = Close File(refnum=w630, error in=w629) -> (path=w623:path, error out=w624:errorcluster)
        n197 = Concatenate Strings(w621, ".txt" ("string")) -> (w619:string)
        n198 = Strip Path(path=w623) -> (stripped path=w626:path)  [unwired: 1 out]
        n199 = Build Path(base path=w626, name or relative path=w619) -> (appended path=w627:path)
        n200 = Copy(8:w624, 10:w627, 11:w623) -> (0:w625:errorcluster)  [unwired: 2 in, 2 out]
        n201 = Delete(path (use dialog)=w623, error in=w625) -> (error out=w622:errorcluster)  [unwired: 3 in, 2 out]
      }
    }
  }
  n202 = while {
    tunnel: [w679] -> w62
    tunnel: [w680] -> w61
    tunnel: ["Use RCVR 8"] -> w63
    shift-right: [w676] -> w64
    shift-left: _ -> [w675]
    shift-right: [w674] -> w65
    shift-left: _ -> [w672]
    tunnel: w38 -> [w671]
    stop <- w677 stop-if-true
    n203 = Unbundle By Name(w671) -> ("shutdown notify"=w673:refnum<notifier>)
    n204 = Get Notifier Status(notifier=w673) -> (current notification=w677:bool)  [unwired: 1 in, 4 out]
    n205 = Compound Arithmetic op=AND("Use RCVR 8", invert w677) -> (w678:bool)
    n206 = case shown="True" w678 {
      tunnel: [w683 w700] -> w680
      tunnel: [w683 w694] -> w679
      tunnel: [w682 "Name of RCVR 8"] -> w676
      tunnel: w675 -> [w682 _]
      tunnel: [w681 w687] -> w674
      tunnel: w672 -> [w681 _]
      tunnel: w671 -> [_ w686]
      frame False {
        w683 = errorcluster {"status"=FALSE, "code"=0, "source"=""} ("error in (no error)")
        n207 = Wait (ms)(milliseconds to wait=u32 1000) -> ()  [unwired: 1 out]
      }
      frame True {
        n208 = call "create RCVR files.vi"("Notifiers"=w686, "Name of RCVR 1"="Name of RCVR 8") -> ("error out"=w688:errorcluster, "refnum out"=w689:refnum<file>, "Name of file out"=w690:string)  [unwired: 7 in]
        n209 = while {
          tunnel: w689 -> [w725]
          tunnel: w688 -> [w724]
          tunnel: [w716] -> w702
          tunnel: [w708] -> w701
          tunnel: [w714] -> w700
          shift-right: [w706] -> w693
          shift-left: w690 -> [w706]
          tunnel: ["COM Port 8"] -> w687
          tunnel: w686 -> [w705]
          tunnel: "Name of RCVR 8" -> [w703]
          stop <- w707 stop-if-true
          n210 = Unbundle By Name("COM Port 8") -> ("COM Port"=w721:refnum<visa-resource-name>, "baud rate"=w720:u32, "data bits"=w719:u16, "parity"=w718:enum16{"None", "Odd", "Even", "Mark", "Space"}, "flow control"=w717:u16)
          n211 = call-poly "VISA Configure Serial Port"("VISA resource name"=w721, "timeout (10sec)"=u32 50, "baud rate (9600)"=w720, "data bits (8)"=w719, "parity (0:none)"=w718, "error in (no error)"=errorcluster {"status"=FALSE, "code"=0, "source"=""}, "flow control (0:none)"=w717) -> ("VISA resource name out"=w723:refnum<visa-resource-name>, "error out"=w722:errorcluster)  [unwired: 7 in]
          n212 = while {
            tunnel: [w737] -> w710
            tunnel: w725 -> [w730]
            tunnel: w724 -> [w729]
            tunnel: w723 -> [w741]
            tunnel: [w735] -> w716
            tunnel: [w734] -> w708
            tunnel: [w733] -> w707
            shift-right: [w738] -> _
            shift-left: _ -> [w739]
            tunnel: w722 -> [w740]
            tunnel: [w736] -> w711
            tunnel: w705 -> [w731]
            tunnel: w703 -> [w726]
            stop <- w732 stop-if-true
            n213 = call "Visa to File.vi"("VISA resource name in"=w741, "Visa Error"=w740, "Array in from shift reg"=w739, "File data refnum"=w730, "File handle Error"=w729, "Notifiers"=w731, "UPDT COM switch"="UPDT COM 8", "Name of RCVR 1"=w726) -> ("End Visa Loop"=w732:bool, "Last 10 RCVR 1"=→"Last 10 RCVR 8":string[], "End File Loop"=w733:bool, "VISA resource name out"=w737:refnum<visa-resource-name>, "Visa error out"=w736:errorcluster, "Array out to shift reg"=w738:string[], "File data refnum out"=w735:refnum<file>, "File Error out"=w734:errorcluster)  [unwired: 4 in]
          }
          n214 = VISA Flush I/O Buffer(VISA resource name=w710, error in (no error)=w711) -> (VISA resource name out=w713:refnum<visa-resource-name>, error out=w712:errorcluster)  [unwired: 1 in]
          n215 = VISA Close(VISA resource name=w713, error in (no error)=w712) -> (error out=w714:errorcluster)
        }
        n216 = Close File(refnum=w702, error in=w701) -> (path=w695:path, error out=w696:errorcluster)
        n217 = Concatenate Strings(w693, ".txt" ("string")) -> (w691:string)
        n218 = Strip Path(path=w695) -> (stripped path=w698:path)  [unwired: 1 out]
        n219 = Build Path(base path=w698, name or relative path=w691) -> (appended path=w699:path)
        n220 = Copy(8:w696, 10:w699, 11:w695) -> (0:w697:errorcluster)  [unwired: 2 in, 2 out]
        n221 = Delete(path (use dialog)=w695, error in=w697) -> (error out=w694:errorcluster)  [unwired: 3 in, 2 out]
      }
    }
  }
  n222 = while {
    tunnel: [w751] -> w55
    tunnel: [w752] -> w56
    tunnel: ["Use RCVR 9"] -> w54
    shift-right: [w748] -> w53
    shift-left: _ -> [w747]
    shift-right: [w746] -> w52
    shift-left: _ -> [w744]
    tunnel: w38 -> [w743]
    stop <- w749 stop-if-true
    n223 = Unbundle By Name(w743) -> ("shutdown notify"=w745:refnum<notifier>)
    n224 = Get Notifier Status(notifier=w745) -> (current notification=w749:bool)  [unwired: 1 in, 4 out]
    n225 = Compound Arithmetic op=AND("Use RCVR 9", invert w749) -> (w750:bool)
    n226 = case shown="True" w750 {
      tunnel: [w755 w772] -> w752
      tunnel: [w755 w766] -> w751
      tunnel: [w754 "Name of RCVR 9"] -> w748
      tunnel: w747 -> [w754 _]
      tunnel: [w753 w759] -> w746
      tunnel: w744 -> [w753 _]
      tunnel: w743 -> [_ w758]
      frame False {
        w755 = errorcluster {"status"=FALSE, "code"=0, "source"=""} ("error in (no error)")
        n227 = Wait (ms)(milliseconds to wait=u32 1000) -> ()  [unwired: 1 out]
      }
      frame True {
        n228 = call "create RCVR files.vi"("Notifiers"=w758, "Name of RCVR 1"="Name of RCVR 9") -> ("error out"=w760:errorcluster, "refnum out"=w761:refnum<file>, "Name of file out"=w762:string)  [unwired: 7 in]
        n229 = while {
          tunnel: w761 -> [w797]
          tunnel: w760 -> [w796]
          tunnel: [w788] -> w774
          tunnel: [w780] -> w773
          tunnel: [w786] -> w772
          shift-right: [w778] -> w765
          shift-left: w762 -> [w778]
          tunnel: ["COM Port 9"] -> w759
          tunnel: w758 -> [w777]
          tunnel: "Name of RCVR 9" -> [w775]
          stop <- w779 stop-if-true
          n230 = Unbundle By Name("COM Port 9") -> ("COM Port"=w793:refnum<visa-resource-name>, "baud rate"=w792:u32, "data bits"=w791:u16, "parity"=w790:enum16{"None", "Odd", "Even", "Mark", "Space"}, "flow control"=w789:u16)
          n231 = call-poly "VISA Configure Serial Port"("VISA resource name"=w793, "timeout (10sec)"=u32 50, "baud rate (9600)"=w792, "data bits (8)"=w791, "parity (0:none)"=w790, "error in (no error)"=errorcluster {"status"=FALSE, "code"=0, "source"=""}, "flow control (0:none)"=w789) -> ("VISA resource name out"=w795:refnum<visa-resource-name>, "error out"=w794:errorcluster)  [unwired: 7 in]
          n232 = while {
            tunnel: [w809] -> w782
            tunnel: w797 -> [w802]
            tunnel: w796 -> [w801]
            tunnel: w795 -> [w813]
            tunnel: [w807] -> w788
            tunnel: [w806] -> w780
            tunnel: [w805] -> w779
            shift-right: [w810] -> _
            shift-left: _ -> [w811]
            tunnel: w794 -> [w812]
            tunnel: [w808] -> w783
            tunnel: w777 -> [w803]
            tunnel: w775 -> [w798]
            stop <- w804 stop-if-true
            n233 = call "Visa to File.vi"("VISA resource name in"=w813, "Visa Error"=w812, "Array in from shift reg"=w811, "File data refnum"=w802, "File handle Error"=w801, "Notifiers"=w803, "UPDT COM switch"="UPDT COM 9", "Name of RCVR 1"=w798) -> ("End Visa Loop"=w804:bool, "Last 10 RCVR 1"=→"Last 10 RCVR 9":string[], "End File Loop"=w805:bool, "VISA resource name out"=w809:refnum<visa-resource-name>, "Visa error out"=w808:errorcluster, "Array out to shift reg"=w810:string[], "File data refnum out"=w807:refnum<file>, "File Error out"=w806:errorcluster)  [unwired: 4 in]
          }
          n234 = VISA Flush I/O Buffer(VISA resource name=w782, error in (no error)=w783) -> (VISA resource name out=w785:refnum<visa-resource-name>, error out=w784:errorcluster)  [unwired: 1 in]
          n235 = VISA Close(VISA resource name=w785, error in (no error)=w784) -> (error out=w786:errorcluster)
        }
        n236 = Close File(refnum=w774, error in=w773) -> (path=w767:path, error out=w768:errorcluster)
        n237 = Concatenate Strings(w765, ".txt" ("string")) -> (w763:string)
        n238 = Strip Path(path=w767) -> (stripped path=w770:path)  [unwired: 1 out]
        n239 = Build Path(base path=w770, name or relative path=w763) -> (appended path=w771:path)
        n240 = Copy(8:w768, 10:w771, 11:w767) -> (0:w769:errorcluster)  [unwired: 2 in, 2 out]
        n241 = Delete(path (use dialog)=w767, error in=w769) -> (error out=w766:errorcluster)  [unwired: 3 in, 2 out]
      }
    }
  }
  n242 = while {
    tunnel: [w823] -> w41
    tunnel: [w824] -> w40
    tunnel: ["Use RCVR 10"] -> w42
    shift-right: [w820] -> w43
    shift-left: _ -> [w819]
    shift-right: [w818] -> w44
    shift-left: _ -> [w816]
    tunnel: w38 -> [w815]
    stop <- w821 stop-if-true
    n243 = Unbundle By Name(w815) -> ("shutdown notify"=w817:refnum<notifier>)
    n244 = Get Notifier Status(notifier=w817) -> (current notification=w821:bool)  [unwired: 1 in, 4 out]
    n245 = Compound Arithmetic op=AND("Use RCVR 10", invert w821) -> (w822:bool)
    n246 = case shown="True" w822 {
      tunnel: [w827 w844] -> w824
      tunnel: [w827 w838] -> w823
      tunnel: [w826 "Name of RCVR 10"] -> w820
      tunnel: w819 -> [w826 _]
      tunnel: [w825 w831] -> w818
      tunnel: w816 -> [w825 _]
      tunnel: w815 -> [_ w830]
      frame False {
        w827 = errorcluster {"status"=FALSE, "code"=0, "source"=""} ("error in (no error)")
        n247 = Wait (ms)(milliseconds to wait=u32 1000) -> ()  [unwired: 1 out]
      }
      frame True {
        n248 = call "create RCVR files.vi"("Notifiers"=w830, "Name of RCVR 1"="Name of RCVR 10") -> ("error out"=w832:errorcluster, "refnum out"=w833:refnum<file>, "Name of file out"=w834:string)  [unwired: 7 in]
        n249 = while {
          tunnel: w833 -> [w869]
          tunnel: w832 -> [w868]
          tunnel: [w860] -> w846
          tunnel: [w852] -> w845
          tunnel: [w858] -> w844
          shift-right: [w850] -> w837
          shift-left: w834 -> [w850]
          tunnel: ["COM Port 10"] -> w831
          tunnel: w830 -> [w849]
          tunnel: "Name of RCVR 10" -> [w847]
          stop <- w851 stop-if-true
          n250 = Unbundle By Name("COM Port 10") -> ("COM Port"=w865:refnum<visa-resource-name>, "baud rate"=w864:u32, "data bits"=w863:u16, "parity"=w862:enum16{"None", "Odd", "Even", "Mark", "Space"}, "flow control"=w861:u16)
          n251 = call-poly "VISA Configure Serial Port"("VISA resource name"=w865, "timeout (10sec)"=u32 50, "baud rate (9600)"=w864, "data bits (8)"=w863, "parity (0:none)"=w862, "error in (no error)"=errorcluster {"status"=FALSE, "code"=0, "source"=""}, "flow control (0:none)"=w861) -> ("VISA resource name out"=w867:refnum<visa-resource-name>, "error out"=w866:errorcluster)  [unwired: 7 in]
          n252 = while {
            tunnel: [w881] -> w854
            tunnel: w869 -> [w874]
            tunnel: w868 -> [w873]
            tunnel: w867 -> [w885]
            tunnel: [w879] -> w860
            tunnel: [w878] -> w852
            tunnel: [w877] -> w851
            shift-right: [w882] -> _
            shift-left: _ -> [w883]
            tunnel: w866 -> [w884]
            tunnel: [w880] -> w855
            tunnel: w849 -> [w875]
            tunnel: w847 -> [w870]
            stop <- w876 stop-if-true
            n253 = call "Visa to File.vi"("VISA resource name in"=w885, "Visa Error"=w884, "Array in from shift reg"=w883, "File data refnum"=w874, "File handle Error"=w873, "Notifiers"=w875, "UPDT COM switch"="UPDT COM 10", "Name of RCVR 1"=w870) -> ("End Visa Loop"=w876:bool, "Last 10 RCVR 1"=→"Last 10 RCVR 10":string[], "End File Loop"=w877:bool, "VISA resource name out"=w881:refnum<visa-resource-name>, "Visa error out"=w880:errorcluster, "Array out to shift reg"=w882:string[], "File data refnum out"=w879:refnum<file>, "File Error out"=w878:errorcluster)  [unwired: 4 in]
          }
          n254 = VISA Flush I/O Buffer(VISA resource name=w854, error in (no error)=w855) -> (VISA resource name out=w857:refnum<visa-resource-name>, error out=w856:errorcluster)  [unwired: 1 in]
          n255 = VISA Close(VISA resource name=w857, error in (no error)=w856) -> (error out=w858:errorcluster)
        }
        n256 = Close File(refnum=w846, error in=w845) -> (path=w839:path, error out=w840:errorcluster)
        n257 = Concatenate Strings(w837, ".txt" ("string")) -> (w835:string)
        n258 = Strip Path(path=w839) -> (stripped path=w842:path)  [unwired: 1 out]
        n259 = Build Path(base path=w842, name or relative path=w835) -> (appended path=w843:path)
        n260 = Copy(8:w840, 10:w843, 11:w839) -> (0:w841:errorcluster)  [unwired: 2 in, 2 out]
        n261 = Delete(path (use dialog)=w839, error in=w841) -> (error out=w838:errorcluster)  [unwired: 3 in, 2 out]
      }
    }
  }
  n262 = while {
    tunnel: [w895] -> w159
    tunnel: [w896] -> w160
    tunnel: ["Use RCVR 1"] -> w140
    shift-right: [w891] -> w139
    shift-left: _ -> [w890]
    shift-right: [w889] -> w138
    shift-left: _ -> [w886]
    tunnel: w38 -> [w887]
    stop <- w893 stop-if-true
    n263 = Unbundle By Name(w887) -> ("shutdown notify"=w888:refnum<notifier>)
    n264 = Get Notifier Status(notifier=w888) -> (current notification=w893:bool)  [unwired: 1 in, 4 out]
    n265 = Compound Arithmetic op=AND("Use RCVR 1", invert w893) -> (w894:bool)
    n266 = case shown="True" w894 {
      tunnel: [w899 w916] -> w896
      tunnel: [w899 w910] -> w895
      tunnel: [w898 "Name of RCVR 1"] -> w891
      tunnel: w890 -> [w898 _]
      tunnel: [w897 w903] -> w889
      tunnel: w886 -> [w897 _]
      tunnel: w887 -> [_ w902]
      frame False {
        w899 = errorcluster {"status"=FALSE, "code"=0, "source"=""} ("error in (no error)")
        n267 = Wait (ms)(milliseconds to wait=u32 1000) -> ()  [unwired: 1 out]
      }
      frame True {
        n268 = call "create RCVR files.vi"("Notifiers"=w902, "Name of RCVR 1"="Name of RCVR 1") -> ("error out"=w904:errorcluster, "refnum out"=w905:refnum<file>, "Name of file out"=w906:string)  [unwired: 7 in]
        n269 = while {
          tunnel: w905 -> [w941]
          tunnel: w904 -> [w940]
          tunnel: [w932] -> w918
          tunnel: [w924] -> w917
          tunnel: [w930] -> w916
          shift-right: [w922] -> w909
          shift-left: w906 -> [w922]
          tunnel: ["COM Port 1"] -> w903
          tunnel: w902 -> [w920]
          tunnel: "Name of RCVR 1" -> [w919]
          stop <- w923 stop-if-true
          n270 = Unbundle By Name("COM Port 1") -> ("COM Port"=w937:refnum<visa-resource-name>, "baud rate"=w936:u32, "data bits"=w935:u16, "parity"=w934:enum16{"None", "Odd", "Even", "Mark", "Space"}, "flow control"=w933:u16)
          n271 = call-poly "VISA Configure Serial Port"("VISA resource name"=w937, "timeout (10sec)"=u32 50, "baud rate (9600)"=w936, "data bits (8)"=w935, "parity (0:none)"=w934, "error in (no error)"=errorcluster {"status"=FALSE, "code"=0, "source"=""}, "flow control (0:none)"=w933) -> ("VISA resource name out"=w939:refnum<visa-resource-name>, "error out"=w938:errorcluster)  [unwired: 7 in]
          n272 = while {
            tunnel: [w952] -> w926
            tunnel: w941 -> [w944]
            tunnel: w940 -> [w943]
            tunnel: w939 -> [w957]
            tunnel: [w949] -> w932
            tunnel: [w948] -> w924
            tunnel: [w947] -> w923
            shift-right: [w953] -> _
            shift-left: _ -> [w954]
            tunnel: w938 -> [w955]
            tunnel: [w950] -> w927
            tunnel: w920 -> [w945]
            tunnel: w919 -> [w942]
            stop <- w946 stop-if-true
            n273 = call "Visa to File.vi"("VISA resource name in"=w957, "Visa Error"=w955, "Array in from shift reg"=w954, "File data refnum"=w944, "File handle Error"=w943, "Notifiers"=w945, "UPDT COM switch"="UPDT COM 1", "Name of RCVR 1"=w942) -> ("End Visa Loop"=w946:bool, "Last 10 RCVR 1"=→"Last 10 RCVR 1":string[], "End File Loop"=w947:bool, "VISA resource name out"=w952:refnum<visa-resource-name>, "Visa error out"=w950:errorcluster, "Array out to shift reg"=w953:string[], "File data refnum out"=w949:refnum<file>, "File Error out"=w948:errorcluster)  [unwired: 4 in]
          }
          n274 = VISA Flush I/O Buffer(VISA resource name=w926, error in (no error)=w927) -> (VISA resource name out=w929:refnum<visa-resource-name>, error out=w928:errorcluster)  [unwired: 1 in]
          n275 = VISA Close(VISA resource name=w929, error in (no error)=w928) -> (error out=w930:errorcluster)
        }
        n276 = Close File(refnum=w918, error in=w917) -> (path=w911:path, error out=w912:errorcluster)
        n277 = Concatenate Strings(w909, ".txt" ("string")) -> (w907:string)
        n278 = Strip Path(path=w911) -> (stripped path=w914:path)  [unwired: 1 out]
        n279 = Build Path(base path=w914, name or relative path=w907) -> (appended path=w915:path)
        n280 = Copy(8:w912, 10:w915, 11:w911) -> (0:w913:errorcluster)  [unwired: 2 in, 2 out]
        n281 = Delete(path (use dialog)=w911, error in=w913) -> (error out=w910:errorcluster)  [unwired: 3 in, 2 out]
      }
    }
  }
  n282 = while {
    shift-right: [w977] -> w170
    shift-left: w181 -> [w979]
    shift-right: [w975] -> w171
    shift-left: w179 -> [w980]
    shift-right: [w973] -> w172
    shift-left: w188 -> [w981]
    shift-right: [w967] -> w173
    shift-left: w191 -> [w982]
    shift-right: [w971] -> _
    shift-left: _ -> [w970]
    tunnel: [w961] -> w135
    tunnel: w38 -> [w960]
    tunnel: [w958] -> w129
    stop <- w966 stop-if-true
    n283 = Bundle By Name(cluster=T7 {"Base File Path"=path "", "Time between samples (seconds)"=5, "Number of hours To Collect before starting new file "=1} ("setup save cluster"), "Time between samples (seconds)"="Time between samples (seconds)", "Base File Path"="Base File Path", "Number of hours To Collect before starting new file"="Number of hours To Collect before starting new file") -> (w961:T7)
    n284 = event shown="[2] Menu Selection (User)" {
      selector: _ -> [_ _ _ _]
      dyn-events: _ -> [_ _ _ _]
      timeout: 50 -> [_ _ _ _]
      tunnel: w982 -> [w1014 w1054 w1061 w1093]
      tunnel: [w1014 w1053 w1062 w1093] -> w972
      tunnel: w981 -> [w1009 w1052 w1060 w1095]
      tunnel: [w1008 w1052 w1060 w1083] -> w974
      tunnel: w980 -> [w1011 w1050 w1058 w1091]
      tunnel: [w1010 w1050 w1058 w1092] -> w976
      tunnel: w979 -> [w1006 w1051 w1059 w1090]
      tunnel: [w1013 w1051 w1059 w1089] -> w978
      tunnel: "Number of hours To Collect before starting new file" -> [w1005 _ _ _]
      tunnel: "Time between samples (seconds)" -> [w1007 _ _ w1080]
      tunnel: "Base File Path" -> [w1012 _ _ w1082]
      tunnel: [w1003 w1048 w1057 w1076] -> w971
      tunnel: w970 -> [w1002 w1048 w1057 w1076]
      tunnel: [w1001 errorcluster {"status"=FALSE, "code"=0, "source"=""} ("error out") errorcluster {"status"=FALSE, "code"=0, "source"=""} ("error out") errorcluster {"status"=FALSE, "code"=0, "source"=""} ("error out")] -> w969
      tunnel: w960 -> [w1000 w1045 w1055 w1071]
      tunnel: [w1000 w1045 w1055 w1071] -> w958
      event Timeout {
        n285 = event-data() -> ()  [unwired: 1 in, 1 out]
        n286 = Unbundle By Name(w1000) -> ("File Path Notify"=w999:refnum<notifier>, "Time smpl notify"=w998:refnum<notifier>, "Update notify"=w997:refnum<notifier>)
        n287 = call "hours between scans.vi"("Number of hours To Collect before starting new file"=w1005, "Input start time"=w1002) -> ("error out"=w1001:errorcluster, "Time has Elapsed"=w1004:bool, "output next start time"=w1003:dbl)  [unwired: 7 in]
        n288 = case shown="True" w1004 {
          tunnel: w1006 -> [w1017 w1039]
          tunnel: [w1017 w1038] -> w1013
          tunnel: w1012 -> [_ w1037]
          tunnel: w1007 -> [_ w1036]
          tunnel: w1011 -> [w1016 w1035]
          tunnel: [w1016 w1034] -> w1010
          tunnel: w1009 -> [w1015 w1027]
          tunnel: [w1015 w1026] -> w1008
          tunnel: w1007 -> [_ w1025]
          tunnel: w999 -> [_ w1020]
          tunnel: w998 -> [_ w1019]
          tunnel: w997 -> [_ w1018]
          frame False {
          }
          frame True {
            n289 = Multiply(x=u32 1000, y=w1025) -> (x*y=w1023:u32)
            n290 = Send Notification(notification=TRUE, notifier=w1018, error in (no error)=w1027) -> (notifier out=w1032:refnum<notifier>, error out=w1031:errorcluster)
            n291 = Add(x=u32 3000 ("milliseconds to wait"), y=w1023) -> (x+y=w1021:u32)
            n292 = while {
              tunnel: w1032 -> [w1041]
              tunnel: w1031 -> [w1042]
              tunnel: [w1042] -> w1029
              tunnel: [w1041] -> w1028
              tunnel: w1021 -> [w1040]
              stop <- TRUE ("stop 2") stop-if-true
              n293 = Wait (ms)(milliseconds to wait=w1040) -> ()  [unwired: 1 out]
            }
            n294 = Send Notification(notification=w1036, notifier=w1019, error in (no error)=w1035) -> (error out=w1034:errorcluster)  [unwired: 1 out]
            n295 = Send Notification(notification=w1037, notifier=w1020, error in (no error)=w1039) -> (error out=w1038:errorcluster)  [unwired: 1 out]
            n296 = Send Notification(notification=FALSE, notifier=w1028, error in (no error)=w1029) -> (error out=w1026:errorcluster)  [unwired: 1 out]
          }
        }
      }
      event "stop": Value Change {
        n297 = event-data() -> ()  [unwired: 1 in, 1 out]
        n298 = Unbundle By Name(w1045) -> ("shutdown notify"=w1046:refnum<notifier>)
        n299 = Send Notification(notification=TRUE, notifier=w1046, error in (no error)=w1054) -> (error out=w1053:errorcluster)  [unwired: 1 out]
        n300 = property on="shutdown blocker" class="Bool (strict)"("Visible"=TRUE) -> ()  [unwired: 2 in, 2 out]
      }
      event Menu Selection (User) {
        n301 = event-data() -> ("ItemTag"=w1063:string)  [unwired: 1 in]
        n302 = case shown="\"ShutDown\"" w1063 {
          tunnel: [w1064 w1070] -> w1062
          tunnel: w1061 -> [w1064 w1069]
          tunnel: w1055 -> [_ w1067]
          frame "0", Default {
            (unwired) FALSE
          }
          frame "ShutDown" {
            n303 = Unbundle By Name(w1067) -> ("shutdown notify"=w1066:refnum<notifier>)
            n304 = Send Notification(notification=TRUE, notifier=w1066, error in (no error)=w1069) -> (error out=w1070:errorcluster)  [unwired: 1 out]
            n305 = property on="shutdown blocker" class="Bool (strict)"("Visible"=TRUE) -> ()  [unwired: 2 in, 2 out]
          }
        }
      }
      event "Update setup": Value Change {
        n306 = event-data() -> ()  [unwired: 1 in, 1 out]
        n307 = Unbundle By Name(w1071) -> ("File Path Notify"=w1072:refnum<notifier>, "Time smpl notify"=w1073:refnum<notifier>, "Update notify"=w1074:refnum<notifier>)
        n308 = Send Notification(notification=TRUE, notifier=w1074, error in (no error)=w1095) -> (notifier out=w1088:refnum<notifier>, error out=w1087:errorcluster)
        n309 = Send Notification(notification=w1082, notifier=w1072, error in (no error)=w1090) -> (error out=w1089:errorcluster)  [unwired: 1 out]
        n310 = Send Notification(notification=w1080, notifier=w1073, error in (no error)=w1091) -> (error out=w1092:errorcluster)  [unwired: 1 out]
        n311 = Multiply(x=u32 1000, y=w1080) -> (x*y=w1081:u32)
        n312 = Add(x=u32 3000 ("milliseconds to wait"), y=w1081) -> (x+y=w1077:u32)
        n313 = while {
          tunnel: w1088 -> [w1097]
          tunnel: w1087 -> [w1098]
          tunnel: [w1098] -> w1085
          tunnel: [w1097] -> w1084
          tunnel: w1077 -> [w1096]
          stop <- TRUE ("stop 2") stop-if-true
          n314 = Wait (ms)(milliseconds to wait=w1096) -> ()  [unwired: 1 out]
        }
        n315 = Send Notification(notification=FALSE, notifier=w1084, error in (no error)=w1085) -> (error out=w1083:errorcluster)  [unwired: 1 out]
      }
    }
    n316 = case shown="Error" w969 {
      frame No Error {
      }
      frame Error {
        n317 = call "Display Message to User15"("Message"="An Error occurred when trying to create new files at time of reset was reached.") -> ()  [unwired: 9 in, 2 out]
      }
    }
    n318 = case shown="Error" w978 {
      selector: w978 -> [w994 _]
      tunnel: [w994 errorcluster {"status"=FALSE, "code"=0, "source"=""} ("error out")] -> w977
      frame No Error {
      }
      frame Error {
        n319 = call "Display Message to User"("Message"="An Error occurred during update of file path. Be sure that the files are saving in the assigned location.") -> ()  [unwired: 9 in, 2 out]
      }
    }
    n320 = case shown="Error" w976 {
      selector: w976 -> [w991 _]
      tunnel: [w991 errorcluster {"status"=FALSE, "code"=0, "source"=""} ("error out")] -> w975
      frame No Error {
      }
      frame Error {
        n321 = call "Display Message to User2"("Message"="An Error occurred during update of the Sample Rate. Be sure that the sample rate of collection is the rate you specified.") -> ()  [unwired: 9 in, 2 out]
      }
    }
    n322 = case shown="Error" w974 {
      selector: w974 -> [w988 _]
      tunnel: [w988 errorcluster {"status"=FALSE, "code"=0, "source"=""} ("error out")] -> w973
      frame No Error {
      }
      frame Error {
        n323 = call "Display Message to User3"("Message"="An Error occurred during the update and create new file. Try the process again and be sure to check that the file locations are correct and the sample rate of collection is correct. If the problem persists close out the software and reopen.") -> ()  [unwired: 9 in, 2 out]
      }
    }
    n324 = case shown="Error" w972 {
      selector: w972 -> [w985 _]
      tunnel: [w985 errorcluster {"status"=FALSE, "code"=0, "source"=""} ("error out")] -> w968
      frame No Error {
      }
      frame Error {
        n325 = call "Display Message to User4"("Message"="An Error occurred during ShutDown.  Try the process again and wait for a minute or two for all processes to end. If the problem persists use the task manager to kill the process COM_2_TXT.exe.  Then change the *.CTSF files that the system was working on to *.TXT extensions recover data and prevent the possible overwrite of data when the software is restarted.") -> ()  [unwired: 9 in, 2 out]
      }
    }
    n326 = Unbundle By Name(w958) -> ("shutdown notify"=w959:refnum<notifier>)
    n327 = Get Notifier Status(notifier=w959, error in (no error)=w968) -> (current notification=w966:bool, error out=w967:errorcluster)  [unwired: 3 out]
  }
  n328 = Bundle By Name(cluster=w14, "Use RCVR 5"=w94, "Name of RCVR 5"=w93, "COM Port 5"=w92) -> (w33:T11)
  n329 = Bundle By Name(cluster=w15, "Use RCVR 4"=w102, "Name of RCVR 4"=w103, "COM Port 4"=w104) -> (w34:T17)
  n330 = Merge Errors(w96, w95) -> (w97:errorcluster)
  n331 = Bundle By Name(cluster=w13, "Use RCVR 6"=w82, "Name of RCVR 6"=w83, "COM Port 6"=w84) -> (w32:T12)
  n332 = Bundle By Name(cluster=w16, "Use RCVR 3"=w114, "Name of RCVR 3"=w113, "COM Port 3"=w112) -> (w35:T10)
  n333 = Merge Errors(w100, w101) -> (w99:errorcluster)
  n334 = Merge Errors(w80, w81) -> (w79:errorcluster)
  n335 = Bundle By Name(cluster=w12, "Use RCVR 7"=w74, "Name of RCVR 7"=w73, "COM Port 7"=w72) -> (w31:T14)
  n336 = Bundle By Name(cluster=w9, "Use RCVR 10"=w42, "Name of RCVR 10"=w43, "COM Port 10"=w44) -> (w28:T13)
  n337 = Merge Errors(w116, w115) -> (w117:errorcluster)
  n338 = Bundle By Name(cluster=w11, "Use RCVR 8"=w63, "Name of RCVR 8"=w64, "COM Port 8"=w65) -> (w30:T16)
  n339 = Bundle By Name(cluster=w17, "Use RCVR 2"=w122, "Name of RCVR 2"=w123, "COM Port 2"=w124) -> (w7:T9)
  n340 = Merge Errors(w76, w75) -> (w77:errorcluster)
  n341 = Merge Errors(w61, w62) -> (w60:errorcluster)
  n342 = Bundle By Name(cluster=w10, "Use RCVR 9"=w54, "Name of RCVR 9"=w53, "COM Port 9"=w52) -> (w29:T15)
  n343 = Merge Errors(w120, w121) -> (w119:errorcluster)
  n344 = Merge Errors(w56, w55) -> (w57:errorcluster)
  n345 = Merge Errors(w40, w41) -> (w39:errorcluster)
  n346 = Bundle By Name(cluster=w18, "Use RCVR 1"=w140, "Name of RCVR 1"=w139, "COM Port 1"=w138) -> (w8:T8)
  n347 = Merge Errors(w160, w159) -> (w161:errorcluster)
  n348 = case shown="Error" w97 {
    selector: w97 -> [w1100 _]
    tunnel: [w1100 errorcluster {"status"=FALSE, "code"=0, "source"=""} ("error out")] -> w88
    frame No Error {
    }
    frame Error {
      n349 = call "Display Message to User10"("Message"="An Error Occurred at RCVR 5 at shutdown.") -> ()  [unwired: 9 in, 2 out]
    }
  }
  n350 = case shown="Error" w99 {
    selector: w99 -> [w1103 _]
    tunnel: [w1103 errorcluster {"status"=FALSE, "code"=0, "source"=""} ("error out")] -> w98
    frame No Error {
    }
    frame Error {
      n351 = call "Display Message to User11"("Message"="An Error Occurred at RCVR 4 at shutdown.") -> ()  [unwired: 9 in, 2 out]
    }
  }
  n352 = case shown="Error" w79 {
    selector: w79 -> [w1106 _]
    tunnel: [w1106 errorcluster {"status"=FALSE, "code"=0, "source"=""} ("error out")] -> w78
    frame No Error {
    }
    frame Error {
      n353 = call "Display Message to User9"("Message"="An Error Occurred at RCVR 6 at shutdown.") -> ()  [unwired: 9 in, 2 out]
    }
  }
  n354 = case shown="Error" w117 {
    selector: w117 -> [w1109 _]
    tunnel: [w1109 errorcluster {"status"=FALSE, "code"=0, "source"=""} ("error out")] -> w111
    frame No Error {
    }
    frame Error {
      n355 = call "Display Message to User12"("Message"="An Error Occurred at RCVR 3 at shutdown.") -> ()  [unwired: 9 in, 2 out]
    }
  }
  n356 = case shown="Error" w77 {
    selector: w77 -> [w1112 _]
    tunnel: [w1112 errorcluster {"status"=FALSE, "code"=0, "source"=""} ("error out")] -> w59
    frame No Error {
    }
    frame Error {
      n357 = call "Display Message to User8"("Message"="An Error Occurred at RCVR 7 at shutdown.") -> ()  [unwired: 9 in, 2 out]
    }
  }
  n358 = case shown="Error" w60 {
    selector: w60 -> [w1115 _]
    tunnel: [w1115 errorcluster {"status"=FALSE, "code"=0, "source"=""} ("error out")] -> w58
    frame No Error {
    }
    frame Error {
      n359 = call "Display Message to User16"("Message"="An Error Occurred at RCVR 8 at shutdown.") -> ()  [unwired: 9 in, 2 out]
    }
  }
  n360 = case shown="Error" w119 {
    selector: w119 -> [w1118 _]
    tunnel: [w1118 errorcluster {"status"=FALSE, "code"=0, "source"=""} ("error out")] -> w118
    frame No Error {
    }
    frame Error {
      n361 = call "Display Message to User13"("Message"="An Error Occurred at RCVR 2 at shutdown.") -> ()  [unwired: 9 in, 2 out]
    }
  }
  n362 = case shown="Error" w57 {
    selector: w57 -> [w1121 _]
    tunnel: [w1121 errorcluster {"status"=FALSE, "code"=0, "source"=""} ("error out")] -> w48
    frame No Error {
    }
    frame Error {
      n363 = call "Display Message to User5"("Message"="An Error Occurred at RCVR 9 at shutdown.") -> ()  [unwired: 9 in, 2 out]
    }
  }
  n364 = case shown="Error" w39 {
    selector: w39 -> [w1124 _]
    tunnel: [w1124 errorcluster {"status"=FALSE, "code"=0, "source"=""} ("error out")] -> w37
    frame No Error {
    }
    frame Error {
      n365 = call "Display Message to User6"("Message"="An Error Occurred at RCVR 10 at shutdown.") -> ()  [unwired: 9 in, 2 out]
    }
  }
  n366 = Merge Errors(w170, w171, w172, w173) -> (w187:errorcluster)
  n367 = case shown="Error" w161 {
    selector: w161 -> [w1127 _]
    tunnel: [w1127 errorcluster {"status"=FALSE, "code"=0, "source"=""} ("error out")] -> w158
    frame No Error {
    }
    frame Error {
      n368 = call "Display Message to User14"("Message"="An Error Occurred at RCVR 1 at shutdown.") -> ()  [unwired: 9 in, 2 out]
    }
  }
  n369 = Merge Errors(w187, w158, w118, w111, w98, w88, w78, w59, w58, w48, w37) -> (w26:errorcluster)
  n370 = Bundle By Name(cluster=T3 {"setup save cluster"={"Base File Path"=path "", "Time between samples (seconds)"=0, "Number of hours To Collect before starting new file "=0}, "RCVR1 Save Cluster"={"Use RCVR 1"=FALSE, "COM Port 1"={"flow control"=0, "COM Port"="", "parity"=enum."None", "data bits"=0, "baud rate"=0}, "Name of RCVR 1"=""}, "RCVR2 Save cluster"={"Use RCVR 2"=FALSE, "COM Port 2"={"flow control"=0, "COM Port"="", "parity"=enum."None", "data bits"=0, "baud rate"=0}, "Name of RCVR 2"=""}, "RCVR3 Save Cluster"={"Use RCVR 3"=FALSE, "Name of RCVR 3"="", "COM Port 3"={"flow control"=0, "COM Port"="", "parity"=enum."None", "data bits"=0, "baud rate"=0}}, "RCVR4 Save Cluster"={"Use RCVR 4"=FALSE, "Name of RCVR 4"="", "COM Port 4"={"flow control"=0, "COM Port"="", "parity"=enum."None", "data bits"=0, "baud rate"=0}}, "RCVR5 Save Cluster"={"Use RCVR 5"=FALSE, "Name of RCVR 5"="", "COM Port 5"={"flow control"=0, "COM Port"="", "parity"=enum."None", "data bits"=0, "baud rate"=0}}, "RCVR6 Save Cluster"={"Use RCVR 6"=FALSE, "Name of RCVR 6"="", "COM Port 6"={"flow control"=0, "COM Port"="", "parity"=enum."None", "data bits"=0, "baud rate"=0}}, "RCVR7 Save Cluster"={"Use RCVR 7"=FALSE, "Name of RCVR 7"="", "COM Port 7"={"flow control"=0, "COM Port"="", "parity"=enum."None", "data bits"=0, "baud rate"=0}}, "RCVR8 Save Cluster"={"Use RCVR 8"=FALSE, "Name of RCVR 8"="", "COM Port 8"={"flow control"=0, "COM Port"="", "parity"=enum."None", "data bits"=0, "baud rate"=0}}, "RCVR9 Save Cluster"={"Use RCVR 9"=FALSE, "Name of RCVR 9"="", "COM Port 9"={"flow control"=0, "COM Port"="", "parity"=enum."None", "data bits"=0, "baud rate"=0}}, "RCVR10 Save Cluster"={"Use RCVR 10"=FALSE, "Name of RCVR 10"="", "COM Port 10"={"flow control"=0, "COM Port"="", "parity"=enum."None", "data bits"=0, "baud rate"=0}}} ("output cluster"), "setup save cluster"=w135, "RCVR1 Save Cluster"=w8, "RCVR2 Save cluster"=w7, "RCVR3 Save Cluster"=w35, "RCVR4 Save Cluster"=w34, "RCVR5 Save Cluster"=w33, "RCVR6 Save Cluster"=w32, "RCVR7 Save Cluster"=w31, "RCVR8 Save Cluster"=w30, "RCVR9 Save Cluster"=w29, "RCVR10 Save Cluster"=w28) -> (w141:T3)
  n371 = call <vilib>:"Get System Directory.vi"("system directory type"=w150) -> ("system directory"=w153:path)  [unwired: 10 in]
  n372 = Build Path(base path=w153, name or relative path="Com2TXT.confg") -> (appended path=w137:path)
  n373 = Write to Binary File(file (use dialog)=w137, data=w141, 9:T5."little-endian" ("byte order (0:big-endian, network order)")) -> (refnum out=w151:refnum<file>, error out=w152:errorcluster)  [unwired: 3 in, 1 out]
  n374 = Close File(refnum=w151, error in=w152) -> (error out=w27:errorcluster)  [unwired: 1 out]
  n375 = Unbundle By Name(w129) -> ("File Path Notify"=w128:refnum<notifier>, "Time smpl notify"=w127:refnum<notifier>, "Update notify"=w126:refnum<notifier>, "shutdown notify"=w125:refnum<notifier>)
  n376 = Merge Errors(w26, w27) -> (w149:errorcluster)
  n377 = call <vilib>:"Simple Error Handler.vi"("error in (no error)"=w149) -> ("error out"=w165:errorcluster)  [unwired: 4 in, 4 out]
  n378 = call <vilib>:"Clear Errors.vi"("error in (no error)"=w165) -> ("error out"=w164:errorcluster)  [unwired: 6 in]
  n379 = Release Notifier(notifier=w125, force destroy? (F)=w166, error in (no error)=w164) -> (error out=w169:errorcluster)  [unwired: 2 out]
  n380 = Release Notifier(notifier=w126, force destroy? (F)=w166, error in (no error)=w169) -> (error out=w168:errorcluster)  [unwired: 2 out]
  n381 = Release Notifier(notifier=w127, force destroy? (F)=w166, error in (no error)=w168) -> (error out=w167:errorcluster)  [unwired: 2 out]
  n382 = Release Notifier(notifier=w128, force destroy? (F)=w166, error in (no error)=w167) -> (error out=w163:errorcluster)  [unwired: 2 out]
  n383 = call <vilib>:"Clear Errors.vi"("error in (no error)"=w163) -> ("error out"=w176:errorcluster)  [unwired: 6 in]
  n384 = property class="App"(error in=w176) -> (error out=w175:errorcluster, "App.Kind"=w174:T18)  [unwired: 1 in, 1 out]
  n385 = case shown="\"Run Time System\"" w174 {
    tunnel: w175 -> [_ _ _ _ _ _ _]
    frame "invalid app kind", Default {
    }
    frame "Development System" {
    }
    frame "Run Time System" {
      n386 = Quit LabVIEW() -> ()  [unwired: 1 in]
    }
    frame "Student Edition" {
    }
    frame "Embedded LabVIEW" {
    }
    frame "Evaluation" {
    }
    frame "Custom" {
    }
  }
